vi "Navigation.vi"(0 "IA State Output in":T14, 1 "Penalty Shoot Out?":bool, 2 "PID gains Vel":T13={"proportional gain (Kc)"=0.6, "integral time (Ti, min)"=0.0, "derivative time (Td, min)"=0.0}, 3 "VelNearBall":dbl=1.0 format="%#_13g", 5 "Test Mode":bool, 6 "PID gains Angle":cluster{"(Kc)":dbl, "(Ki)":dbl, "(Kd)":dbl}={"(Kc)"=0.0, "(Ki)"=0.3, "(Kd)"=1.0}, 7 "a1":dbl=10.0, 8 "PID gains Lateral":cluster{"(Kc)":dbl, "(Ki)":dbl, "(Kd)":dbl}={"(Kc)"=2.0, "(Ki)"=0.0, "(Kd)"=0.3}, 9 "a3":dbl=15.0, 10 "Old GoTo Params":T12={"PID gains Angle GoTo"={"(Kc)"=3.0, "(Ki)"=0.0, "(Kd)"=2.0}, "PID gains XY GoTo"={"(Kc)"=3.0, "(Ki)"=0.0, "(Kd)"=2.0}, "Max Params GoTo"={"Max output XY"=3.0, "MaxOutput Angle"=0.0}}, 11 "GoTo Navigation":bool, 12 "Debug":bool, 13 "output inc":dbl, 14 "output xy":dbl, 15 "output angle":dbl) -> (4 "IA State Output out":T14)   [LabVIEW 2023]
uses:
  Vision_class/Old vision/SSL Detection Frame Simple Estimator Cameras VelCmd Folder/Core/AI Input.ctl
  Vision_class/Old vision/Controls/AI Robot.ctl
  Vision_class/Old vision/Controls/Functions Enum.ctl
  Controls/estimatives.ctl
  Vision_class/Old vision/Controls/AttackerStates.ctl
  Vision_class/Old vision/Controls/PathDests.ctl
  Vision_class/Old vision/Controls/PathDest.ctl
  VSSNavigation/VSSAttackerStates.ctl
  Robot_class/robotKickToStates.ctl
  Robot_class/roles.ctl
  <vilib>/Analysis/Matrix/Datatypes/RealMatrix.ctl
  driveMode.ctl
  Vision_class/Old vision/SSL Detection Frame Simple Estimator Cameras VelCmd Folder/Core/AI Ball.ctl
  Vision_class/Old vision/SSL Detection Frame Simple Estimator Cameras VelCmd Folder/Core/Field Size.ctl
  Vision_class/Old vision/SSL Detection Frame Simple Estimator Cameras VelCmd Folder/Core/AI Judge.ctl
  Communication_class/Paths/MessageAI_State Folder/Intel/Command Enum.ctl
  Vision_class/Old vision/SSL Detection Frame Simple Estimator Cameras VelCmd Folder/Util/Events/Events.ctl
  Utilities_class/Utilities.lvclass
  <vilib>/Analysis/Matrix/NI_Matrix.lvlib
panel:
  in  "Robot":T1={"id"=0, "function"=enum."Attacker", "x"=0.0, "y"=0.0, "orientation"=0.0, "v_tangent"=0.0, "v_normal"=0.0, "v_ang"=0.0, "kick_x"=0.0, "kick_z"=0.0, "dribble"=FALSE, "Timestamp"=timestamp(0 s since 1904-01-01), "estimatives"={"est_v_tangent"=0.0, "est_v_normal"=0.0, "est_vx"=0.0, "est_vy"=0.0, "Pos Robot Est"=[], "est_v_ang"=0.0}, "dest_x_kick"=0.0, "dest_y_kick"=0.0, "Gap Coord"=[], "States"=enum."GoToTangent", "Path "=[], "Path  Smooth"=[], "Dest"=[], "vx_desired"=0.0, "vy_desired"=0.0, "slowBehavior"=FALSE, "VSSStates"=enum."Pass", "robotKickState"=enum."none", "role"=enum."DefenderArea", "x_k|k"=[], "driveMode"=enum."Fast"}
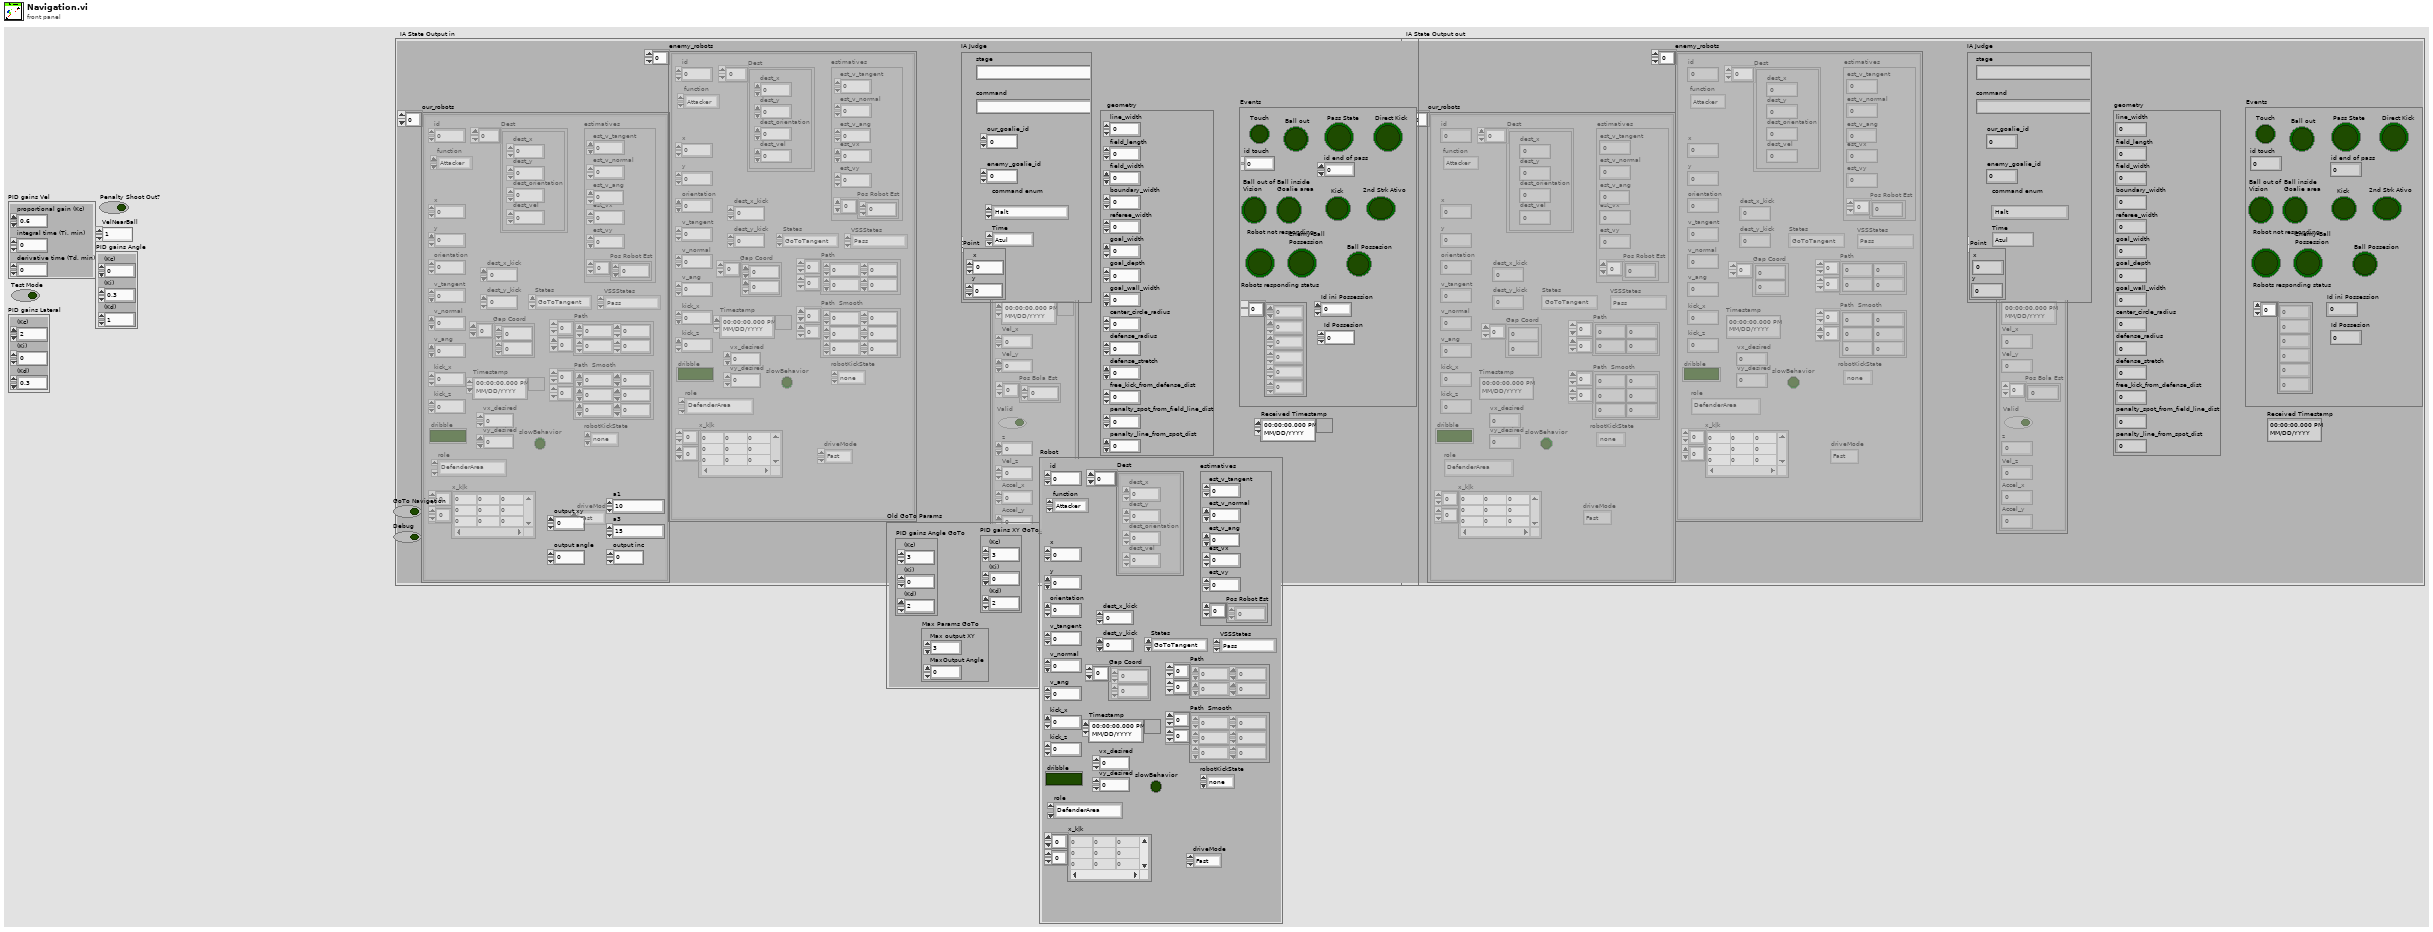
[diagram p1: front panel]
types:
  T1 = typedef "AI Robot.ctl" = cluster{"id":u32, "function":T2, "x":dbl, "y":dbl, "orientation":dbl, "v_tangent":dbl, "v_normal":dbl, "v_ang":dbl, "kick_x":dbl, "kick_z":dbl, "dribble":bool, "Timestamp":timestamp, "estimatives":T3, "dest_x_kick":dbl, "dest_y_kick":dbl, "Gap Coord":dbl[], "States":T4, "Path ":dbl[][], "Path  Smooth":dbl[][], "Dest":T5, "vx_desired":dbl, "vy_desired":dbl, "slowBehavior":bool, "VSSStates":T7, "robotKickState":T8, "role":T9, "x_k|k":T10, "driveMode":T11}
  T2 = typedef "Functions Enum.ctl" = enum16{"2nd Striker", "Attacker", "Goalie", "Defender", "Striker", "Goto 0", "Dummy", "Kicker", "ZigZag 0", "ZigZag 1", "ZigZag 2", "ZigZag 3", "ZigZag 4", "ZigZag 5", "ZigZag 6", "ZigZag 7", "ZigZag 8"}
  T3 = typedef "estimatives.ctl" = cluster{"est_v_tangent":dbl, "est_v_normal":dbl, "est_vx":dbl, "est_vy":dbl, "Pos Robot Est":dbl[], "est_v_ang":dbl}
  T4 = typedef "AttackerStates.ctl" = enum16{"Pass", "GoToTangent", "BallGetting", "GoToKick", ""}
  T5 = typedef "PathDests.ctl" = T6[]
  T6 = typedef "PathDest.ctl" = cluster{"dest_x":dbl, "dest_y":dbl, "dest_orientation":dbl, "dest_vel":dbl}
  T7 = typedef "VSSAttackerStates.ctl" = enum16{"Pass", "GoToTangent", "BallGetting", "GoToKick", "Rotate anti-clockwise", "Rotate Clockwise", ""}
  T8 = typedef "robotKickToStates.ctl" = enum16{"shootFromDirect", "avoidCollideBall", "goToBackBall", "none", "walk", "turn", "oldKickToShoot", "oldKickToGoToBackBall", "shoot"}
  T9 = typedef "roles.ctl" = enum16{"SimpleBallPlacement", "BallPlacementAllyPasser", "BallPlacementAllyReceiver", "BallPlacementEnemy", "5Robots5th", "PassBestReceiver", "5Robots4th", "5Robots3rd", "5Robots2nd", "5Robots1st", "PassBestRobot", "WaitPass", "ABCThirdKicker", "ABCFirstKicker", "ABCSecondKicker", "Tabler", "TableFinalizer", "PrepareRollToPassRoller", "PrepareRollToPassReceiver", "SimplePassRoll", "SimplePassRollReceiver", "PenaltyDefense", "PreparePassReceiver 2", "PreparePassReceiver 1", "PassObserver", "Timeout", "Goto", "ZigZag", "None", "BallOutOfField", "DefenderArea", "Duelist", "AttackerStop", "FollowAttacker", "KeeperRole", "KickPenalty", "AttackerAimGoal", "AttackerBlock", "Marker", "Halt", "Shoot", "PassKicker", "PassReceiver", "TestRole", "PenaltyAttacker", "PrimaryAttackerRole", "SupportAttackerRole"}
  T10 = typedef "NI_Matrix.lvlib/RealMatrix.ctl" = dbl[][]
  T11 = typedef "driveMode.ctl" = enum16{"Fast", "SafeDrive"}
  T12 = cluster{"PID gains Angle GoTo":cluster{"(Kc)":dbl, "(Ki)":dbl, "(Kd)":dbl}, "PID gains XY GoTo":cluster{"(Kc)":dbl, "(Ki)":dbl, "(Kd)":dbl}, "Max Params GoTo":cluster{"Max output XY":dbl, "MaxOutput Angle":dbl}}
  T13 = cluster{"proportional gain (Kc)":dbl, "integral time (Ti, min)":dbl, "derivative time (Td, min)":dbl}
  T14 = typedef "AI Input.ctl" = cluster{"our_robots":T1[], "enemy_robots":T1[], "balls":T15[], "geometry":T16, "IA Judge":T17, "Received Timestamp":timestamp, "Events":T19}
  T15 = typedef "AI Ball.ctl" = cluster{"x":dbl, "y":dbl, "timestamp":timestamp, "Vel_x":dbl, "Vel_y":dbl, "Pos Bola Est":dbl[], "Valid":bool, "z":dbl, "Vel_z":dbl, "Accel_x":dbl, "Accel_y":dbl}
  T16 = typedef "Field Size.ctl" = cluster{"line_width":u32, "field_length":u32, "field_width":u32, "boundary_width":u32, "referee_width":u32, "goal_width":u32, "goal_depth":u32, "goal_wall_width":u32, "center_circle_radius":u32, "defense_radius":u32, "defense_stretch":u32, "free_kick_from_defense_dist":u32, "penalty_spot_from_field_line_dist":u32, "penalty_line_from_spot_dist":u32}
  T17 = typedef "AI Judge.ctl" = cluster{"stage":string, "command":string, "our_goalie_id":dbl, "enemy_goalie_id":dbl, "command enum":T18, "Time":enum16{"Azul", "Amarelo"}, "Point":cluster{"x":sgl, "y":sgl}}
  T18 = typedef "Command Enum.ctl" = enum16{"Halt", "Stop", "Force Start", "PKA Normal Start", "Prepare Kickoff Ally", "PKE Normal Start", "Prepare Kickoff Enemy", "Prepare Penalty Ally", "PPA Normal Start", "Prepare Penalty Enemy", "PPE Normal Start", "Direct Free Enemy", "Direct Free Ally", "Indirect Free Enemy", "Indirect Free Ally", "Timeout Enemy", "Timeout Ally", "Goal Enemy", "Goal Ally", "Ball Placement Enemy", "Ball Placement Ally", "Normal Half Time", "Extra Time Break", "Extra Half Time", "None", "Post Game"}
  T19 = typedef "Events.ctl" = cluster{"Touch":bool, "Ball out":bool, "id touch":dbl, "Ball out of \nVision":bool, "Ball inside \nGoalie area":bool, "Robot not responding":bool, "Robots responding status":dbl[], "Enemy Ball \nPossession":bool, "Pass State":bool, "id end of pass":dbl, "Kick":bool, "Id ini Possession":dbl, "Ball Possesion":bool, "Id Possesion":dbl, "Direct Kick":bool, "2nd Strk Ativo":bool}
  T20 = cluster{"Max output XY":dbl, "MaxOutput Angle":dbl}
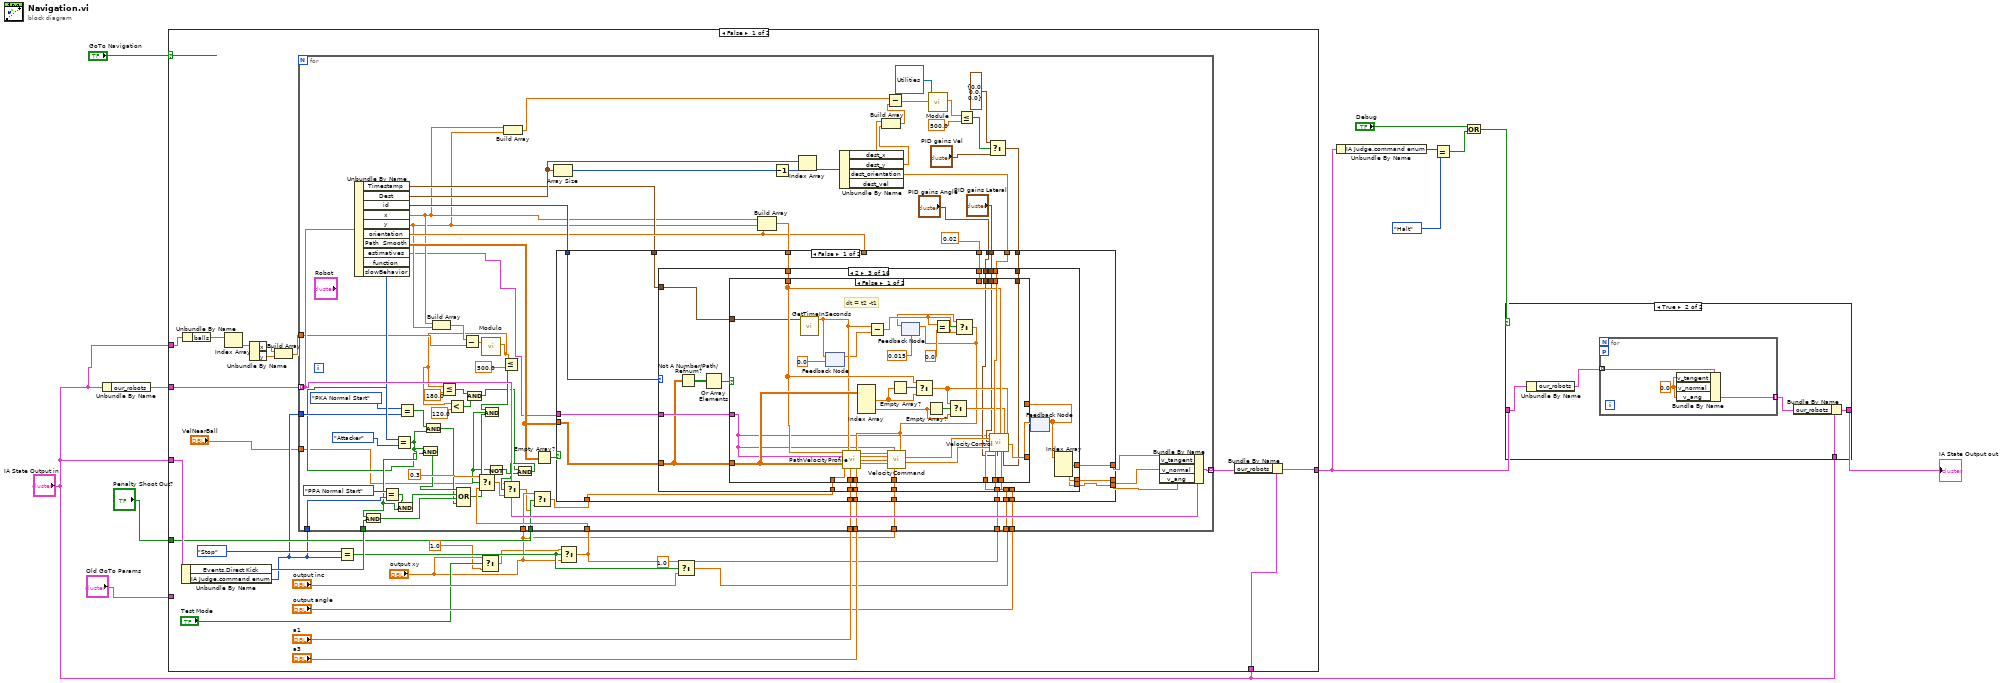
[diagram p0: block diagram]
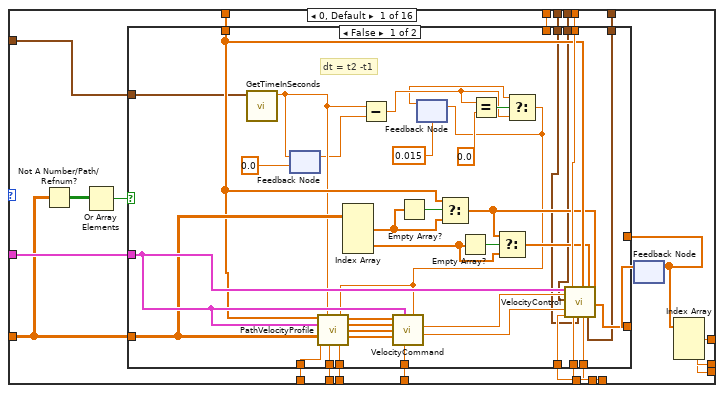
[diagram p2: hidden frame]
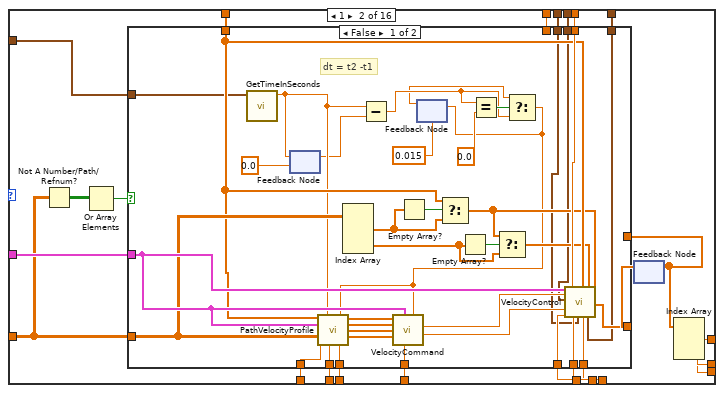
[diagram p4: hidden frame]
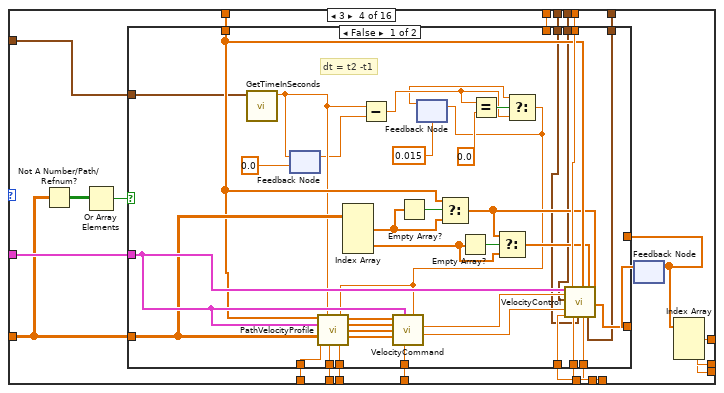
[diagram p7: hidden frame]
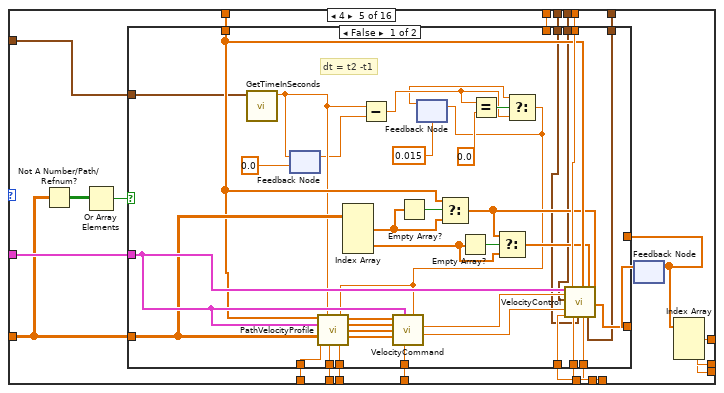
[diagram p9: hidden frame]
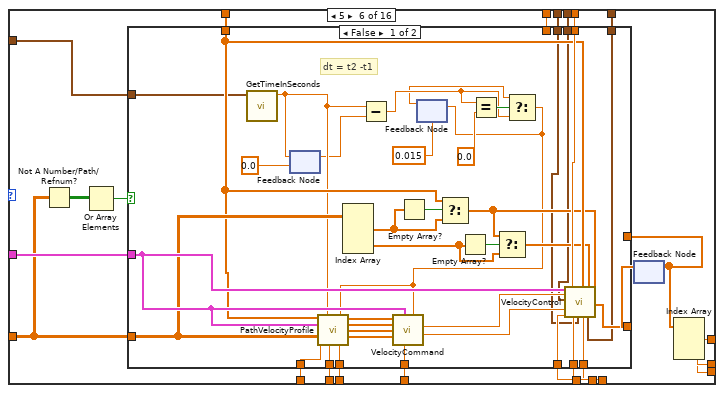
[diagram p11: hidden frame]
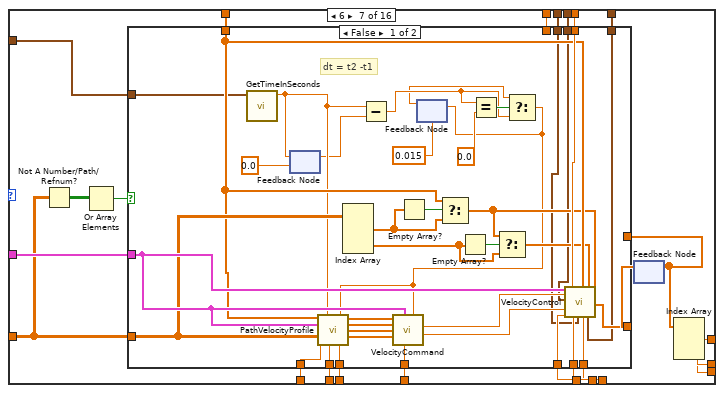
[diagram p13: hidden frame]
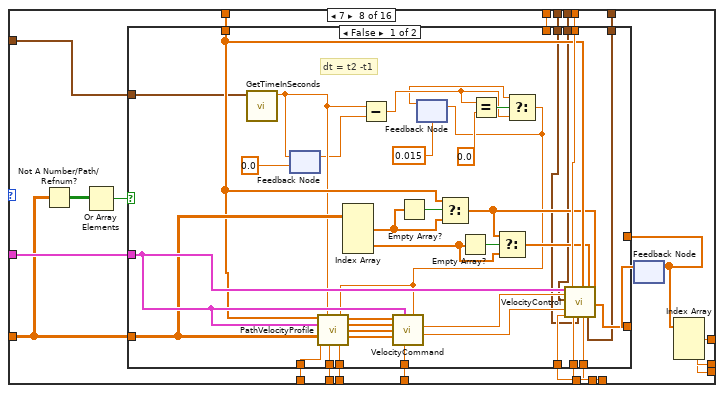
[diagram p15: hidden frame]
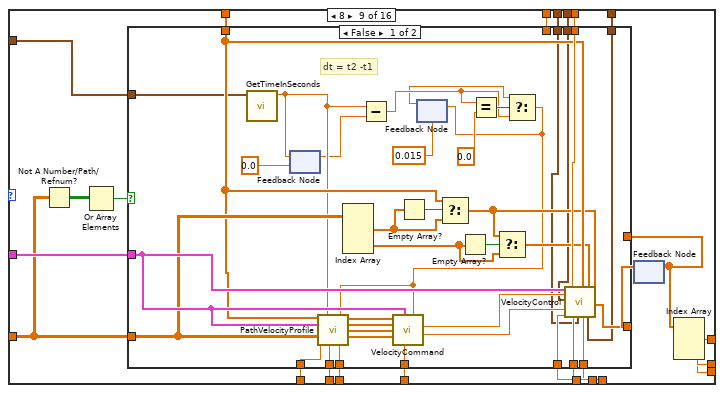
[diagram p17: hidden frame]
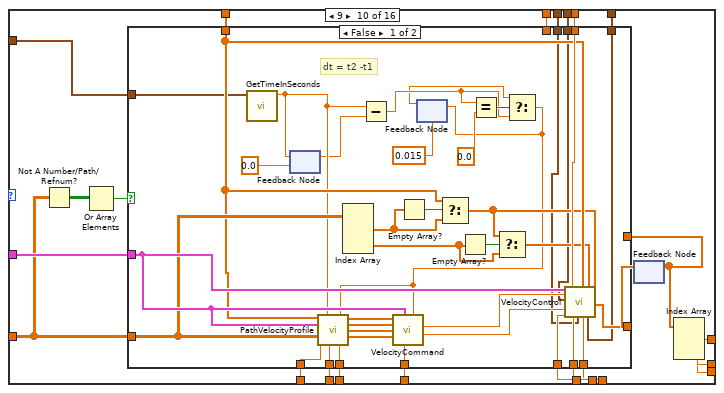
[diagram p19: hidden frame]
diagram:
  n1 = Unbundle By Name("IA State Output in") -> ("our_robots"=w12:T1[])
  n2 = case shown="False" "GoTo Navigation" {
    tunnel: w12 -> [w40 _]
    tunnel: [w37 w1121] -> w9
    tunnel: "IA State Output in" -> [w33 w1119]
    tunnel: "IA State Output in" -> [w38 _]
    tunnel: "IA State Output in" -> [w22 _]
    tunnel: "Penalty Shoot Out?" -> [w19 _]
    tunnel: "Old GoTo Params" -> [_ w1116]
    frame False {
      n3 = Unbundle By Name(w33) -> ("Events.Direct Kick"=w27:bool, "IA Judge.command enum"=w14:T18)
      n4 = Unbundle By Name(w22) -> ("balls"=w26:T15[])
      n5 = Index Array(array=w26) -> (element=w25:T15)  [unwired: 1 in]
      n6 = Unbundle By Name(w25) -> ("x"=w24:dbl, "y"=w23:dbl)
      n7 = Build Array(w24, w23) -> (w21:dbl[])
      n8 = Equal?(x=Command_Enum."Stop", y=w14) -> (x = y?=w20:bool)
      n9 = Select(t="output xy", s="Test Mode", f=1.0 ("t")) -> (s? t:f=w15:dbl)
      n10 = Select(t=w15, s=w20, f="output xy") -> (s? t:f=w31:dbl)
      n11 = Select(t=1.0, s=w20, f="output inc") -> (s? t:f=w29:dbl)
      n12 = for {
        tunnel: w40 -> [w118] mode=indexing
        tunnel: [w117] -> w39 mode=indexing
        tunnel: w31 -> [w96]
        tunnel: "a1" -> [w107]
        tunnel: "a3" -> [w106]
        tunnel: w29 -> [w102]
        tunnel: "output angle" -> [w101]
        tunnel: w31 -> [w100]
        tunnel: w14 -> [w94]
        tunnel: w27 -> [w88]
        tunnel: w14 -> [w86]
        tunnel: w21 -> [w77]
        tunnel: w19 -> [w74]
        tunnel: "output xy" -> [w73]
        tunnel: "output xy" -> [w58]
        tunnel: "VelNearBall" -> [w49]
        n13 = Unbundle By Name(w118) -> ("Timestamp"=w98:timestamp, "Dest"=w116:T5, "id"=w109:u32, "x"=w71:dbl, "y"=w70:dbl, "orientation"=w105:dbl, "Path  Smooth"=w110:dbl[][], "estimatives"=w46:T3, "function"=w87:T2, "slowBehavior"=w56:bool)
        n14 = Equal?(x=Command_Enum."PPA Normal Start", y=w94) -> (x = y?=w91:bool)
        n15 = Equal?(x=w87, y=Functions_Enum."Attacker") -> (x = y?=w83:bool)
        n16 = And(x=w83, y=w88) -> (x .and. y?=w89:bool)
        n17 = And(x=w91, y=w83) -> (x .and. y?=w90:bool)
        n18 = Equal?(x=Command_Enum."PKA Normal Start", y=w86) -> (x = y?=w84:bool)
        n19 = And(x=w83, y=w56) -> (x .and. y?=w92:bool)
        n20 = And(x=w84, y=w83) -> (x .and. y?=w82:bool)
        n21 = Build Array(w71, w70) -> (w78:dbl[])
        n22 = Compound Arithmetic op=OR(w92, w90, w89, w82) -> (w79:bool)
        n23 = Subtract(x=w78, y=w77) -> (x-y=w76:dbl[])
        n24 = call "Modulo.vi"("2D vector"=w76) -> ("Modulo"=w45:dbl)  [unwired: 10 in]
        n25 = Less Or Equal?(x=w45, y=180.0) -> (x <= y?=w43:bool)
        n26 = Less?(x=w45, y=120.0) -> (x < y?=w44:bool)
        n27 = And(x=w43, y=w44) -> (x .and. y?=w42:bool)
        n28 = Less Or Equal?(x=w45, y=500.0) -> (x <= y?=w80:bool)
        n29 = And(x=w80, y=w79) -> (x .and. y?=w54:bool)
        n30 = Select(t=0.3, s=w54, f=w96) -> (s? t:f=w51:dbl)
        n31 = Not(x=w54) -> (.not. x?=w53:bool)
        n32 = Build Array(w71, w70) -> (w66:dbl[])
        n33 = And(x=w42, y=w53) -> (x .and. y?=w52:bool)
        n34 = Select(t=w49, s=w52, f=w51) -> (s? t:f=w50:dbl)
        n35 = Select(t=w73, s=w74, f=w50) -> (s? t:f=w72:dbl)
        n36 = Empty Array?(array=w110) -> (empty?=w111:bool)
        n37 = Array Size(array=w116) -> (size(s)=w115:i32)
        n38 = Build Array(w71, w70, w105) -> (w108:dbl[])
        n39 = Decrement(x=w115) -> (x-1=w114:i32)
        n40 = Index Array(array=w116, index=w114) -> (element=w113:T6)
        n41 = Unbundle By Name(w113) -> ("dest_x"=w69:dbl, "dest_y"=w68:dbl, "dest_orientation"=w112:dbl)  [unwired: 1 out]
        n42 = Build Array(w69, w68) -> (w67:dbl[])
        n43 = Subtract(x=w66, y=w67) -> (x-y=w65:dbl[])
        n44 = call "Module.vi"("2D vector"=w65, "Utilities in"=refnum<class "Utilities.lvclass"> refnum) -> ("Modulo"=w63:dbl)  [unwired: 7 in, 2 out]
        n45 = Less Or Equal?(x=w63, y=500.0) -> (x <= y?=w61:bool)
        n46 = Select(t=T13 {"proportional gain (Kc)"=0.0, "integral time (Ti, min)"=0.0, "derivative time (Td, min)"=0.0}, s=w61, f="PID gains Vel") -> (s? t:f=w60:T13)
        n47 = case shown="False" w111 {
          tunnel: [w128 w1115] -> w104
          tunnel: [w127 w1115] -> w103
          tunnel: [w126 w1115] -> w99
          tunnel: w109 -> [w124 _]
          tunnel: w110 -> [w130 _]
          tunnel: w112 -> [w131 _]
          tunnel: w108 -> [w129 _]
          tunnel: w46 -> [w132 _]
          tunnel: w72 -> [w138 _]
          tunnel: w107 -> [w137 _]
          tunnel: w106 -> [w136 _]
          tunnel: w105 -> [_ _]
          tunnel: w102 -> [w135 _]
          tunnel: w101 -> [w134 _]
          tunnel: w100 -> [w133 _]
          tunnel: w98 -> [w125 _]
          tunnel: 0.02 -> [w123 _]
          tunnel: w60 -> [w122 _]
          tunnel: w58 -> [w121 _]
          tunnel: "PID gains Angle" -> [w120 _]
          tunnel: "PID gains Lateral" -> [w119 _]
          frame False {
            n48 = case shown="2" w124 {
              tunnel: w138 -> [w161 w222 w283 w344 w405 w466 w527 w588 w649 w710 w771 w832 w893 w954 w1015 w1076]
              tunnel: w137 -> [w160 w221 w282 w343 w404 w465 w526 w587 w648 w709 w770 w831 w892 w953 w1014 w1075]
              tunnel: w136 -> [w159 w220 w281 w342 w403 w464 w525 w586 w647 w708 w769 w830 w891 w952 w1013 w1074]
              tunnel: w135 -> [w158 w219 w280 w341 w402 w463 w524 w585 w646 w707 w768 w829 w890 w951 w1012 w1073]
              tunnel: w134 -> [w157 w218 w279 w340 w401 w462 w523 w584 w645 w706 w767 w828 w889 w950 w1011 w1072]
              tunnel: w133 -> [w156 w217 w278 w339 w400 w461 w522 w583 w644 w705 w766 w827 w888 w949 w1010 w1071]
              tunnel: w132 -> [w155 w216 w277 w338 w399 w460 w521 w582 w643 w704 w765 w826 w887 w948 w1009 w1070]
              tunnel: w131 -> [w154 w215 w276 w337 w398 w459 w520 w581 w642 w703 w764 w825 w886 w947 w1008 w1069]
              tunnel: w130 -> [w146 w207 w268 w329 w390 w451 w512 w573 w634 w695 w756 w817 w878 w939 w1000 w1061]
              tunnel: w129 -> [w153 w214 w275 w336 w397 w458 w519 w580 w641 w702 w763 w824 w885 w946 w1007 w1068]
              tunnel: [w152 w213 w274 w335 w396 w457 w518 w579 w640 w701 w762 w823 w884 w945 w1006 w1067] -> w128
              tunnel: [w151 w212 w273 w334 w395 w456 w517 w578 w639 w700 w761 w822 w883 w944 w1005 w1066] -> w127
              tunnel: [w150 w211 w272 w333 w394 w455 w516 w577 w638 w699 w760 w821 w882 w943 w1004 w1065] -> w126
              tunnel: w125 -> [w149 w210 w271 w332 w393 w454 w515 w576 w637 w698 w759 w820 w881 w942 w1003 w1064]
              tunnel: w123 -> [w143 w204 w265 w326 w387 w448 w509 w570 w631 w692 w753 w814 w875 w936 w997 w1058]
              tunnel: w122 -> [w142 w203 w264 w325 w386 w447 w508 w569 w630 w691 w752 w813 w874 w935 w996 w1057]
              tunnel: w121 -> [w141 w202 w263 w324 w385 w446 w507 w568 w629 w690 w751 w812 w873 w934 w995 w1056]
              tunnel: w120 -> [w140 w201 w262 w323 w384 w445 w506 w567 w628 w689 w750 w811 w872 w933 w994 w1055]
              tunnel: w119 -> [w139 w200 w261 w322 w383 w444 w505 w566 w627 w688 w749 w810 w871 w932 w993 w1054]
              frame 0, Default {
                n49 = Not A Number/Path/Refnum?(number/path/refnum=w146) -> (NaN/Path/Refnum?=w145:bool[][])
                n50 = Or Array Elements(Boolean array=w145) -> (logical OR=w144:bool)
                n51 = feedback #1() -> (w147:dbl[])  [unwired: 1 in]
                n52 = case shown="False" w144 {
                  tunnel: w161 -> [w198 _]
                  tunnel: w160 -> [w197 _]
                  tunnel: w159 -> [w196 _]
                  tunnel: w158 -> [w195 _]
                  tunnel: w157 -> [w194 _]
                  tunnel: w156 -> [w193 _]
                  tunnel: w155 -> [w192 _]
                  tunnel: w154 -> [w191 _]
                  tunnel: w146 -> [w190 _]
                  tunnel: w153 -> [w189 _]
                  tunnel: [w188 w199] -> w148
                  tunnel: w149 -> [w175 _]
                  tunnel: w147 -> [_ w199]
                  tunnel: w143 -> [_ _]
                  tunnel: w142 -> [w166 _]
                  tunnel: w141 -> [w164 _]
                  tunnel: w140 -> [w163 _]
                  tunnel: w139 -> [w162 _]
                  frame False {
                    # "dt = t2 -t1"
                    n53 = call "GetTimeInSeconds.vi"("Timestamp"=w175) -> ("Numeric"=w169:dbl)  [unwired: 10 in]
                    n54 = feedback-in #2(w169) -> ()
                    n55 = feedback #2(0.0 ("Numeric")) -> (w168:dbl)
                    n56 = Index Array(array=w190) -> (element #1=w177:dbl[], element #2=w180:dbl[])  [unwired: 4 in]
                    n57 = Subtract(x=w169, y=w168) -> (x-y=w171:dbl)
                    n58 = Empty Array?(array=w177) -> (empty?=w178:bool)
                    n59 = feedback #3(0.015 ("Numeric")) -> (w170:dbl)
                    n60 = Select(t=w189, s=w178, f=w177) -> (s? t:f=w176:dbl[])
                    n61 = Empty Array?(array=w180) -> (empty?=w181:bool)
                    n62 = Equal?(x=w171, y=0.0) -> (x = y?=w174:bool)
                    n63 = Select(t=w176, s=w181, f=w180) -> (s? t:f=w179:dbl[])
                    n64 = Select(t=w170, s=w174, f=w171) -> (s? t:f=w165:dbl)
                    n65 = call "PathVelocityProfile.vi"("Pose"=w189, "time"=w169, "intervalo"=w165, "estimatives"=w192, "Path  Smooth"=w190, "V_max"=w198, "Accel"=w197, "DesAccel"=w196) -> ("Time X"=w187:dbl[], "Velocities X"=w186:dbl[], "Time Y"=w185:dbl[], "Velocities Y"=w184:dbl[])  [unwired: 4 in]
                    n66 = call "VelocityCommand.vi"("intervalo"=w165, "MaxOutputXY"=w164, "estimatives"=w192, "Velocities Y"=w184, "Time Y"=w185, "Velocities X"=w186, "Time X"=w187) -> ("Vy"=w183:dbl, "Vx"=w182:dbl)  [unwired: 3 in]
                    n67 = feedback-in #3(w165) -> ()
                    n68 = call "VelocityControl.vi"("estimatives"=w192, "Vx"=w182, "PID Gains lateral"=w162, "Vy"=w183, "output xy"=w193, "Dest_orientation"=w191, "output inc"=w195, "PID Gains Angle"=w163, "Position"=w189, "output angle"=w194, "Waypoint 1"=w179, "PID gains Vel"=w166, "Waypoint 0"=w176) -> ("Output Velocity"=w188:dbl[])  [unwired: 6 in]
                  }
                  frame True {
                  }
                }
                n69 = feedback-in #1(w148) -> ()
                n70 = Index Array(array=w147) -> (element #1=w152:dbl, element #2=w151:dbl, element #3=w150:dbl)  [unwired: 3 in]
              }
              frame 1 {
                n71 = Not A Number/Path/Refnum?(number/path/refnum=w207) -> (NaN/Path/Refnum?=w206:bool[][])
                n72 = Or Array Elements(Boolean array=w206) -> (logical OR=w205:bool)
                n73 = feedback #4() -> (w208:dbl[])  [unwired: 1 in]
                n74 = case shown="False" w205 {
                  tunnel: w222 -> [w259 _]
                  tunnel: w221 -> [w258 _]
                  tunnel: w220 -> [w257 _]
                  tunnel: w219 -> [w256 _]
                  tunnel: w218 -> [w255 _]
                  tunnel: w217 -> [w254 _]
                  tunnel: w216 -> [w253 _]
                  tunnel: w215 -> [w252 _]
                  tunnel: w207 -> [w251 _]
                  tunnel: w214 -> [w250 _]
                  tunnel: [w249 w260] -> w209
                  tunnel: w210 -> [w236 _]
                  tunnel: w208 -> [_ w260]
                  tunnel: w204 -> [_ _]
                  tunnel: w203 -> [w227 _]
                  tunnel: w202 -> [w225 _]
                  tunnel: w201 -> [w224 _]
                  tunnel: w200 -> [w223 _]
                  frame False {
                    # "dt = t2 -t1"
                    n75 = call "GetTimeInSeconds.vi"("Timestamp"=w236) -> ("Numeric"=w230:dbl)  [unwired: 10 in]
                    n76 = feedback-in #5(w230) -> ()
                    n77 = feedback #5(0.0 ("Numeric")) -> (w229:dbl)
                    n78 = Index Array(array=w251) -> (element #1=w238:dbl[], element #2=w241:dbl[])  [unwired: 4 in]
                    n79 = Subtract(x=w230, y=w229) -> (x-y=w232:dbl)
                    n80 = Empty Array?(array=w238) -> (empty?=w239:bool)
                    n81 = feedback #6(0.015 ("Numeric")) -> (w231:dbl)
                    n82 = Select(t=w250, s=w239, f=w238) -> (s? t:f=w237:dbl[])
                    n83 = Empty Array?(array=w241) -> (empty?=w242:bool)
                    n84 = Equal?(x=w232, y=0.0) -> (x = y?=w235:bool)
                    n85 = Select(t=w237, s=w242, f=w241) -> (s? t:f=w240:dbl[])
                    n86 = Select(t=w231, s=w235, f=w232) -> (s? t:f=w226:dbl)
                    n87 = call "PathVelocityProfile.vi"("Pose"=w250, "time"=w230, "intervalo"=w226, "estimatives"=w253, "Path  Smooth"=w251, "V_max"=w259, "Accel"=w258, "DesAccel"=w257) -> ("Time X"=w248:dbl[], "Velocities X"=w247:dbl[], "Time Y"=w246:dbl[], "Velocities Y"=w245:dbl[])  [unwired: 4 in]
                    n88 = call "VelocityCommand.vi"("intervalo"=w226, "MaxOutputXY"=w225, "estimatives"=w253, "Velocities Y"=w245, "Time Y"=w246, "Velocities X"=w247, "Time X"=w248) -> ("Vy"=w244:dbl, "Vx"=w243:dbl)  [unwired: 3 in]
                    n89 = feedback-in #6(w226) -> ()
                    n90 = call "VelocityControl.vi"("estimatives"=w253, "Vx"=w243, "PID Gains lateral"=w223, "Vy"=w244, "output xy"=w254, "Dest_orientation"=w252, "output inc"=w256, "PID Gains Angle"=w224, "Position"=w250, "output angle"=w255, "Waypoint 1"=w240, "PID gains Vel"=w227, "Waypoint 0"=w237) -> ("Output Velocity"=w249:dbl[])  [unwired: 6 in]
                  }
                  frame True {
                  }
                }
                n91 = feedback-in #4(w209) -> ()
                n92 = Index Array(array=w208) -> (element #1=w213:dbl, element #2=w212:dbl, element #3=w211:dbl)  [unwired: 3 in]
              }
              frame 2 {
                n93 = Not A Number/Path/Refnum?(number/path/refnum=w268) -> (NaN/Path/Refnum?=w267:bool[][])
                n94 = Or Array Elements(Boolean array=w267) -> (logical OR=w266:bool)
                n95 = feedback #7() -> (w269:dbl[])  [unwired: 1 in]
                n96 = case shown="False" w266 {
                  tunnel: w283 -> [w320 _]
                  tunnel: w282 -> [w319 _]
                  tunnel: w281 -> [w318 _]
                  tunnel: w280 -> [w317 _]
                  tunnel: w279 -> [w316 _]
                  tunnel: w278 -> [w315 _]
                  tunnel: w277 -> [w284 _]
                  tunnel: w276 -> [w314 _]
                  tunnel: w268 -> [w313 _]
                  tunnel: w275 -> [w312 _]
                  tunnel: [w311 w321] -> w270
                  tunnel: w271 -> [w298 _]
                  tunnel: w269 -> [_ w321]
                  tunnel: w265 -> [_ _]
                  tunnel: w264 -> [w289 _]
                  tunnel: w263 -> [w287 _]
                  tunnel: w262 -> [w286 _]
                  tunnel: w261 -> [w285 _]
                  frame False {
                    # "dt = t2 -t1"
                    n97 = call "GetTimeInSeconds.vi"("Timestamp"=w298) -> ("Numeric"=w292:dbl)  [unwired: 10 in]
                    n98 = feedback-in #8(w292) -> ()
                    n99 = feedback #8(0.0 ("Numeric")) -> (w291:dbl)
                    n100 = Index Array(array=w313) -> (element #1=w300:dbl[], element #2=w303:dbl[])  [unwired: 4 in]
                    n101 = Subtract(x=w292, y=w291) -> (x-y=w294:dbl)
                    n102 = Empty Array?(array=w300) -> (empty?=w301:bool)
                    n103 = feedback #9(0.015 ("Numeric")) -> (w293:dbl)
                    n104 = Select(t=w312, s=w301, f=w300) -> (s? t:f=w299:dbl[])
                    n105 = Empty Array?(array=w303) -> (empty?=w304:bool)
                    n106 = Equal?(x=w294, y=0.0) -> (x = y?=w297:bool)
                    n107 = Select(t=w299, s=w304, f=w303) -> (s? t:f=w302:dbl[])
                    n108 = Select(t=w293, s=w297, f=w294) -> (s? t:f=w288:dbl)
                    n109 = call "PathVelocityProfile.vi"("Pose"=w312, "time"=w292, "intervalo"=w288, "estimatives"=w284, "Path  Smooth"=w313, "V_max"=w320, "Accel"=w319, "DesAccel"=w318) -> ("Time X"=w310:dbl[], "Velocities X"=w309:dbl[], "Time Y"=w308:dbl[], "Velocities Y"=w307:dbl[])  [unwired: 4 in]
                    n110 = call "VelocityCommand.vi"("intervalo"=w288, "MaxOutputXY"=w287, "estimatives"=w284, "Velocities Y"=w307, "Time Y"=w308, "Velocities X"=w309, "Time X"=w310) -> ("Vy"=w306:dbl, "Vx"=w305:dbl)  [unwired: 3 in]
                    n111 = feedback-in #9(w288) -> ()
                    n112 = call "VelocityControl.vi"("estimatives"=w284, "Vx"=w305, "PID Gains lateral"=w285, "Vy"=w306, "output xy"=w315, "Dest_orientation"=w314, "output inc"=w317, "PID Gains Angle"=w286, "Position"=w312, "output angle"=w316, "Waypoint 1"=w302, "PID gains Vel"=w289, "Waypoint 0"=w299) -> ("Output Velocity"=w311:dbl[])  [unwired: 6 in]
                  }
                  frame True {
                  }
                }
                n113 = feedback-in #7(w270) -> ()
                n114 = Index Array(array=w269) -> (element #1=w274:dbl, element #2=w273:dbl, element #3=w272:dbl)  [unwired: 3 in]
              }
              frame 3 {
                n115 = Not A Number/Path/Refnum?(number/path/refnum=w329) -> (NaN/Path/Refnum?=w328:bool[][])
                n116 = Or Array Elements(Boolean array=w328) -> (logical OR=w327:bool)
                n117 = feedback #10() -> (w330:dbl[])  [unwired: 1 in]
                n118 = case shown="False" w327 {
                  tunnel: w344 -> [w381 _]
                  tunnel: w343 -> [w380 _]
                  tunnel: w342 -> [w379 _]
                  tunnel: w341 -> [w378 _]
                  tunnel: w340 -> [w377 _]
                  tunnel: w339 -> [w376 _]
                  tunnel: w338 -> [w375 _]
                  tunnel: w337 -> [w374 _]
                  tunnel: w329 -> [w373 _]
                  tunnel: w336 -> [w372 _]
                  tunnel: [w371 w382] -> w331
                  tunnel: w332 -> [w358 _]
                  tunnel: w330 -> [_ w382]
                  tunnel: w326 -> [_ _]
                  tunnel: w325 -> [w349 _]
                  tunnel: w324 -> [w347 _]
                  tunnel: w323 -> [w346 _]
                  tunnel: w322 -> [w345 _]
                  frame False {
                    # "dt = t2 -t1"
                    n119 = call "GetTimeInSeconds.vi"("Timestamp"=w358) -> ("Numeric"=w352:dbl)  [unwired: 10 in]
                    n120 = feedback-in #11(w352) -> ()
                    n121 = feedback #11(0.0 ("Numeric")) -> (w351:dbl)
                    n122 = Index Array(array=w373) -> (element #1=w360:dbl[], element #2=w363:dbl[])  [unwired: 4 in]
                    n123 = Subtract(x=w352, y=w351) -> (x-y=w354:dbl)
                    n124 = Empty Array?(array=w360) -> (empty?=w361:bool)
                    n125 = feedback #12(0.015 ("Numeric")) -> (w353:dbl)
                    n126 = Select(t=w372, s=w361, f=w360) -> (s? t:f=w359:dbl[])
                    n127 = Empty Array?(array=w363) -> (empty?=w364:bool)
                    n128 = Equal?(x=w354, y=0.0) -> (x = y?=w357:bool)
                    n129 = Select(t=w359, s=w364, f=w363) -> (s? t:f=w362:dbl[])
                    n130 = Select(t=w353, s=w357, f=w354) -> (s? t:f=w348:dbl)
                    n131 = call "PathVelocityProfile.vi"("Pose"=w372, "time"=w352, "intervalo"=w348, "estimatives"=w375, "Path  Smooth"=w373, "V_max"=w381, "Accel"=w380, "DesAccel"=w379) -> ("Time X"=w370:dbl[], "Velocities X"=w369:dbl[], "Time Y"=w368:dbl[], "Velocities Y"=w367:dbl[])  [unwired: 4 in]
                    n132 = call "VelocityCommand.vi"("intervalo"=w348, "MaxOutputXY"=w347, "estimatives"=w375, "Velocities Y"=w367, "Time Y"=w368, "Velocities X"=w369, "Time X"=w370) -> ("Vy"=w366:dbl, "Vx"=w365:dbl)  [unwired: 3 in]
                    n133 = feedback-in #12(w348) -> ()
                    n134 = call "VelocityControl.vi"("estimatives"=w375, "Vx"=w365, "PID Gains lateral"=w345, "Vy"=w366, "output xy"=w376, "Dest_orientation"=w374, "output inc"=w378, "PID Gains Angle"=w346, "Position"=w372, "output angle"=w377, "Waypoint 1"=w362, "PID gains Vel"=w349, "Waypoint 0"=w359) -> ("Output Velocity"=w371:dbl[])  [unwired: 6 in]
                  }
                  frame True {
                  }
                }
                n135 = feedback-in #10(w331) -> ()
                n136 = Index Array(array=w330) -> (element #1=w335:dbl, element #2=w334:dbl, element #3=w333:dbl)  [unwired: 3 in]
              }
              frame 4 {
                n137 = Not A Number/Path/Refnum?(number/path/refnum=w390) -> (NaN/Path/Refnum?=w389:bool[][])
                n138 = Or Array Elements(Boolean array=w389) -> (logical OR=w388:bool)
                n139 = feedback #13() -> (w391:dbl[])  [unwired: 1 in]
                n140 = case shown="False" w388 {
                  tunnel: w405 -> [w442 _]
                  tunnel: w404 -> [w441 _]
                  tunnel: w403 -> [w440 _]
                  tunnel: w402 -> [w439 _]
                  tunnel: w401 -> [w438 _]
                  tunnel: w400 -> [w437 _]
                  tunnel: w399 -> [w436 _]
                  tunnel: w398 -> [w435 _]
                  tunnel: w390 -> [w434 _]
                  tunnel: w397 -> [w433 _]
                  tunnel: [w432 w443] -> w392
                  tunnel: w393 -> [w419 _]
                  tunnel: w391 -> [_ w443]
                  tunnel: w387 -> [_ _]
                  tunnel: w386 -> [w410 _]
                  tunnel: w385 -> [w408 _]
                  tunnel: w384 -> [w407 _]
                  tunnel: w383 -> [w406 _]
                  frame False {
                    # "dt = t2 -t1"
                    n141 = call "GetTimeInSeconds.vi"("Timestamp"=w419) -> ("Numeric"=w413:dbl)  [unwired: 10 in]
                    n142 = feedback-in #14(w413) -> ()
                    n143 = feedback #14(0.0 ("Numeric")) -> (w412:dbl)
                    n144 = Index Array(array=w434) -> (element #1=w421:dbl[], element #2=w424:dbl[])  [unwired: 4 in]
                    n145 = Subtract(x=w413, y=w412) -> (x-y=w415:dbl)
                    n146 = Empty Array?(array=w421) -> (empty?=w422:bool)
                    n147 = feedback #15(0.015 ("Numeric")) -> (w414:dbl)
                    n148 = Select(t=w433, s=w422, f=w421) -> (s? t:f=w420:dbl[])
                    n149 = Empty Array?(array=w424) -> (empty?=w425:bool)
                    n150 = Equal?(x=w415, y=0.0) -> (x = y?=w418:bool)
                    n151 = Select(t=w420, s=w425, f=w424) -> (s? t:f=w423:dbl[])
                    n152 = Select(t=w414, s=w418, f=w415) -> (s? t:f=w409:dbl)
                    n153 = call "PathVelocityProfile.vi"("Pose"=w433, "time"=w413, "intervalo"=w409, "estimatives"=w436, "Path  Smooth"=w434, "V_max"=w442, "Accel"=w441, "DesAccel"=w440) -> ("Time X"=w431:dbl[], "Velocities X"=w430:dbl[], "Time Y"=w429:dbl[], "Velocities Y"=w428:dbl[])  [unwired: 4 in]
                    n154 = call "VelocityCommand.vi"("intervalo"=w409, "MaxOutputXY"=w408, "estimatives"=w436, "Velocities Y"=w428, "Time Y"=w429, "Velocities X"=w430, "Time X"=w431) -> ("Vy"=w427:dbl, "Vx"=w426:dbl)  [unwired: 3 in]
                    n155 = feedback-in #15(w409) -> ()
                    n156 = call "VelocityControl.vi"("estimatives"=w436, "Vx"=w426, "PID Gains lateral"=w406, "Vy"=w427, "output xy"=w437, "Dest_orientation"=w435, "output inc"=w439, "PID Gains Angle"=w407, "Position"=w433, "output angle"=w438, "Waypoint 1"=w423, "PID gains Vel"=w410, "Waypoint 0"=w420) -> ("Output Velocity"=w432:dbl[])  [unwired: 6 in]
                  }
                  frame True {
                  }
                }
                n157 = feedback-in #13(w392) -> ()
                n158 = Index Array(array=w391) -> (element #1=w396:dbl, element #2=w395:dbl, element #3=w394:dbl)  [unwired: 3 in]
              }
              frame 5 {
                n159 = Not A Number/Path/Refnum?(number/path/refnum=w451) -> (NaN/Path/Refnum?=w450:bool[][])
                n160 = Or Array Elements(Boolean array=w450) -> (logical OR=w449:bool)
                n161 = feedback #16() -> (w452:dbl[])  [unwired: 1 in]
                n162 = case shown="False" w449 {
                  tunnel: w466 -> [w503 _]
                  tunnel: w465 -> [w502 _]
                  tunnel: w464 -> [w501 _]
                  tunnel: w463 -> [w500 _]
                  tunnel: w462 -> [w499 _]
                  tunnel: w461 -> [w498 _]
                  tunnel: w460 -> [w497 _]
                  tunnel: w459 -> [w496 _]
                  tunnel: w451 -> [w495 _]
                  tunnel: w458 -> [w494 _]
                  tunnel: [w493 w504] -> w453
                  tunnel: w454 -> [w480 _]
                  tunnel: w452 -> [_ w504]
                  tunnel: w448 -> [_ _]
                  tunnel: w447 -> [w471 _]
                  tunnel: w446 -> [w469 _]
                  tunnel: w445 -> [w468 _]
                  tunnel: w444 -> [w467 _]
                  frame False {
                    # "dt = t2 -t1"
                    n163 = call "GetTimeInSeconds.vi"("Timestamp"=w480) -> ("Numeric"=w474:dbl)  [unwired: 10 in]
                    n164 = feedback-in #17(w474) -> ()
                    n165 = feedback #17(0.0 ("Numeric")) -> (w473:dbl)
                    n166 = Index Array(array=w495) -> (element #1=w482:dbl[], element #2=w485:dbl[])  [unwired: 4 in]
                    n167 = Subtract(x=w474, y=w473) -> (x-y=w476:dbl)
                    n168 = Empty Array?(array=w482) -> (empty?=w483:bool)
                    n169 = feedback #18(0.015 ("Numeric")) -> (w475:dbl)
                    n170 = Select(t=w494, s=w483, f=w482) -> (s? t:f=w481:dbl[])
                    n171 = Empty Array?(array=w485) -> (empty?=w486:bool)
                    n172 = Equal?(x=w476, y=0.0) -> (x = y?=w479:bool)
                    n173 = Select(t=w481, s=w486, f=w485) -> (s? t:f=w484:dbl[])
                    n174 = Select(t=w475, s=w479, f=w476) -> (s? t:f=w470:dbl)
                    n175 = call "PathVelocityProfile.vi"("Pose"=w494, "time"=w474, "intervalo"=w470, "estimatives"=w497, "Path  Smooth"=w495, "V_max"=w503, "Accel"=w502, "DesAccel"=w501) -> ("Time X"=w492:dbl[], "Velocities X"=w491:dbl[], "Time Y"=w490:dbl[], "Velocities Y"=w489:dbl[])  [unwired: 4 in]
                    n176 = call "VelocityCommand.vi"("intervalo"=w470, "MaxOutputXY"=w469, "estimatives"=w497, "Velocities Y"=w489, "Time Y"=w490, "Velocities X"=w491, "Time X"=w492) -> ("Vy"=w488:dbl, "Vx"=w487:dbl)  [unwired: 3 in]
                    n177 = feedback-in #18(w470) -> ()
                    n178 = call "VelocityControl.vi"("estimatives"=w497, "Vx"=w487, "PID Gains lateral"=w467, "Vy"=w488, "output xy"=w498, "Dest_orientation"=w496, "output inc"=w500, "PID Gains Angle"=w468, "Position"=w494, "output angle"=w499, "Waypoint 1"=w484, "PID gains Vel"=w471, "Waypoint 0"=w481) -> ("Output Velocity"=w493:dbl[])  [unwired: 6 in]
                  }
                  frame True {
                  }
                }
                n179 = feedback-in #16(w453) -> ()
                n180 = Index Array(array=w452) -> (element #1=w457:dbl, element #2=w456:dbl, element #3=w455:dbl)  [unwired: 3 in]
              }
              frame 6 {
                n181 = Not A Number/Path/Refnum?(number/path/refnum=w512) -> (NaN/Path/Refnum?=w511:bool[][])
                n182 = Or Array Elements(Boolean array=w511) -> (logical OR=w510:bool)
                n183 = feedback #19() -> (w513:dbl[])  [unwired: 1 in]
                n184 = case shown="False" w510 {
                  tunnel: w527 -> [w564 _]
                  tunnel: w526 -> [w563 _]
                  tunnel: w525 -> [w562 _]
                  tunnel: w524 -> [w561 _]
                  tunnel: w523 -> [w560 _]
                  tunnel: w522 -> [w559 _]
                  tunnel: w521 -> [w558 _]
                  tunnel: w520 -> [w557 _]
                  tunnel: w512 -> [w556 _]
                  tunnel: w519 -> [w555 _]
                  tunnel: [w554 w565] -> w514
                  tunnel: w515 -> [w541 _]
                  tunnel: w513 -> [_ w565]
                  tunnel: w509 -> [_ _]
                  tunnel: w508 -> [w532 _]
                  tunnel: w507 -> [w530 _]
                  tunnel: w506 -> [w529 _]
                  tunnel: w505 -> [w528 _]
                  frame False {
                    # "dt = t2 -t1"
                    n185 = call "GetTimeInSeconds.vi"("Timestamp"=w541) -> ("Numeric"=w535:dbl)  [unwired: 10 in]
                    n186 = feedback-in #20(w535) -> ()
                    n187 = feedback #20(0.0 ("Numeric")) -> (w534:dbl)
                    n188 = Index Array(array=w556) -> (element #1=w543:dbl[], element #2=w546:dbl[])  [unwired: 4 in]
                    n189 = Subtract(x=w535, y=w534) -> (x-y=w537:dbl)
                    n190 = Empty Array?(array=w543) -> (empty?=w544:bool)
                    n191 = feedback #21(0.015 ("Numeric")) -> (w536:dbl)
                    n192 = Select(t=w555, s=w544, f=w543) -> (s? t:f=w542:dbl[])
                    n193 = Empty Array?(array=w546) -> (empty?=w547:bool)
                    n194 = Equal?(x=w537, y=0.0) -> (x = y?=w540:bool)
                    n195 = Select(t=w542, s=w547, f=w546) -> (s? t:f=w545:dbl[])
                    n196 = Select(t=w536, s=w540, f=w537) -> (s? t:f=w531:dbl)
                    n197 = call "PathVelocityProfile.vi"("Pose"=w555, "time"=w535, "intervalo"=w531, "estimatives"=w558, "Path  Smooth"=w556, "V_max"=w564, "Accel"=w563, "DesAccel"=w562) -> ("Time X"=w553:dbl[], "Velocities X"=w552:dbl[], "Time Y"=w551:dbl[], "Velocities Y"=w550:dbl[])  [unwired: 4 in]
                    n198 = call "VelocityCommand.vi"("intervalo"=w531, "MaxOutputXY"=w530, "estimatives"=w558, "Velocities Y"=w550, "Time Y"=w551, "Velocities X"=w552, "Time X"=w553) -> ("Vy"=w549:dbl, "Vx"=w548:dbl)  [unwired: 3 in]
                    n199 = feedback-in #21(w531) -> ()
                    n200 = call "VelocityControl.vi"("estimatives"=w558, "Vx"=w548, "PID Gains lateral"=w528, "Vy"=w549, "output xy"=w559, "Dest_orientation"=w557, "output inc"=w561, "PID Gains Angle"=w529, "Position"=w555, "output angle"=w560, "Waypoint 1"=w545, "PID gains Vel"=w532, "Waypoint 0"=w542) -> ("Output Velocity"=w554:dbl[])  [unwired: 6 in]
                  }
                  frame True {
                  }
                }
                n201 = feedback-in #19(w514) -> ()
                n202 = Index Array(array=w513) -> (element #1=w518:dbl, element #2=w517:dbl, element #3=w516:dbl)  [unwired: 3 in]
              }
              frame 7 {
                n203 = Not A Number/Path/Refnum?(number/path/refnum=w573) -> (NaN/Path/Refnum?=w572:bool[][])
                n204 = Or Array Elements(Boolean array=w572) -> (logical OR=w571:bool)
                n205 = feedback #22() -> (w574:dbl[])  [unwired: 1 in]
                n206 = case shown="False" w571 {
                  tunnel: w588 -> [w625 _]
                  tunnel: w587 -> [w624 _]
                  tunnel: w586 -> [w623 _]
                  tunnel: w585 -> [w622 _]
                  tunnel: w584 -> [w621 _]
                  tunnel: w583 -> [w620 _]
                  tunnel: w582 -> [w619 _]
                  tunnel: w581 -> [w618 _]
                  tunnel: w573 -> [w617 _]
                  tunnel: w580 -> [w616 _]
                  tunnel: [w615 w626] -> w575
                  tunnel: w576 -> [w602 _]
                  tunnel: w574 -> [_ w626]
                  tunnel: w570 -> [_ _]
                  tunnel: w569 -> [w593 _]
                  tunnel: w568 -> [w591 _]
                  tunnel: w567 -> [w590 _]
                  tunnel: w566 -> [w589 _]
                  frame False {
                    # "dt = t2 -t1"
                    n207 = call "GetTimeInSeconds.vi"("Timestamp"=w602) -> ("Numeric"=w596:dbl)  [unwired: 10 in]
                    n208 = feedback-in #23(w596) -> ()
                    n209 = feedback #23(0.0 ("Numeric")) -> (w595:dbl)
                    n210 = Index Array(array=w617) -> (element #1=w604:dbl[], element #2=w607:dbl[])  [unwired: 4 in]
                    n211 = Subtract(x=w596, y=w595) -> (x-y=w598:dbl)
                    n212 = Empty Array?(array=w604) -> (empty?=w605:bool)
                    n213 = feedback #24(0.015 ("Numeric")) -> (w597:dbl)
                    n214 = Select(t=w616, s=w605, f=w604) -> (s? t:f=w603:dbl[])
                    n215 = Empty Array?(array=w607) -> (empty?=w608:bool)
                    n216 = Equal?(x=w598, y=0.0) -> (x = y?=w601:bool)
                    n217 = Select(t=w603, s=w608, f=w607) -> (s? t:f=w606:dbl[])
                    n218 = Select(t=w597, s=w601, f=w598) -> (s? t:f=w592:dbl)
                    n219 = call "PathVelocityProfile.vi"("Pose"=w616, "time"=w596, "intervalo"=w592, "estimatives"=w619, "Path  Smooth"=w617, "V_max"=w625, "Accel"=w624, "DesAccel"=w623) -> ("Time X"=w614:dbl[], "Velocities X"=w613:dbl[], "Time Y"=w612:dbl[], "Velocities Y"=w611:dbl[])  [unwired: 4 in]
                    n220 = call "VelocityCommand.vi"("intervalo"=w592, "MaxOutputXY"=w591, "estimatives"=w619, "Velocities Y"=w611, "Time Y"=w612, "Velocities X"=w613, "Time X"=w614) -> ("Vy"=w610:dbl, "Vx"=w609:dbl)  [unwired: 3 in]
                    n221 = feedback-in #24(w592) -> ()
                    n222 = call "VelocityControl.vi"("estimatives"=w619, "Vx"=w609, "PID Gains lateral"=w589, "Vy"=w610, "output xy"=w620, "Dest_orientation"=w618, "output inc"=w622, "PID Gains Angle"=w590, "Position"=w616, "output angle"=w621, "Waypoint 1"=w606, "PID gains Vel"=w593, "Waypoint 0"=w603) -> ("Output Velocity"=w615:dbl[])  [unwired: 6 in]
                  }
                  frame True {
                  }
                }
                n223 = feedback-in #22(w575) -> ()
                n224 = Index Array(array=w574) -> (element #1=w579:dbl, element #2=w578:dbl, element #3=w577:dbl)  [unwired: 3 in]
              }
              frame 8 {
                n225 = Not A Number/Path/Refnum?(number/path/refnum=w634) -> (NaN/Path/Refnum?=w633:bool[][])
                n226 = Or Array Elements(Boolean array=w633) -> (logical OR=w632:bool)
                n227 = feedback #25() -> (w635:dbl[])  [unwired: 1 in]
                n228 = case shown="False" w632 {
                  tunnel: w649 -> [w686 _]
                  tunnel: w648 -> [w685 _]
                  tunnel: w647 -> [w684 _]
                  tunnel: w646 -> [w683 _]
                  tunnel: w645 -> [w682 _]
                  tunnel: w644 -> [w681 _]
                  tunnel: w643 -> [w680 _]
                  tunnel: w642 -> [w679 _]
                  tunnel: w634 -> [w678 _]
                  tunnel: w641 -> [w677 _]
                  tunnel: [w676 w687] -> w636
                  tunnel: w637 -> [w663 _]
                  tunnel: w635 -> [_ w687]
                  tunnel: w631 -> [_ _]
                  tunnel: w630 -> [w654 _]
                  tunnel: w629 -> [w652 _]
                  tunnel: w628 -> [w651 _]
                  tunnel: w627 -> [w650 _]
                  frame False {
                    # "dt = t2 -t1"
                    n229 = call "GetTimeInSeconds.vi"("Timestamp"=w663) -> ("Numeric"=w657:dbl)  [unwired: 10 in]
                    n230 = feedback-in #26(w657) -> ()
                    n231 = feedback #26(0.0 ("Numeric")) -> (w656:dbl)
                    n232 = Index Array(array=w678) -> (element #1=w665:dbl[], element #2=w668:dbl[])  [unwired: 4 in]
                    n233 = Subtract(x=w657, y=w656) -> (x-y=w659:dbl)
                    n234 = Empty Array?(array=w665) -> (empty?=w666:bool)
                    n235 = feedback #27(0.015 ("Numeric")) -> (w658:dbl)
                    n236 = Select(t=w677, s=w666, f=w665) -> (s? t:f=w664:dbl[])
                    n237 = Empty Array?(array=w668) -> (empty?=w669:bool)
                    n238 = Equal?(x=w659, y=0.0) -> (x = y?=w662:bool)
                    n239 = Select(t=w664, s=w669, f=w668) -> (s? t:f=w667:dbl[])
                    n240 = Select(t=w658, s=w662, f=w659) -> (s? t:f=w653:dbl)
                    n241 = call "PathVelocityProfile.vi"("Pose"=w677, "time"=w657, "intervalo"=w653, "estimatives"=w680, "Path  Smooth"=w678, "V_max"=w686, "Accel"=w685, "DesAccel"=w684) -> ("Time X"=w675:dbl[], "Velocities X"=w674:dbl[], "Time Y"=w673:dbl[], "Velocities Y"=w672:dbl[])  [unwired: 4 in]
                    n242 = call "VelocityCommand.vi"("intervalo"=w653, "MaxOutputXY"=w652, "estimatives"=w680, "Velocities Y"=w672, "Time Y"=w673, "Velocities X"=w674, "Time X"=w675) -> ("Vy"=w671:dbl, "Vx"=w670:dbl)  [unwired: 3 in]
                    n243 = feedback-in #27(w653) -> ()
                    n244 = call "VelocityControl.vi"("estimatives"=w680, "Vx"=w670, "PID Gains lateral"=w650, "Vy"=w671, "output xy"=w681, "Dest_orientation"=w679, "output inc"=w683, "PID Gains Angle"=w651, "Position"=w677, "output angle"=w682, "Waypoint 1"=w667, "PID gains Vel"=w654, "Waypoint 0"=w664) -> ("Output Velocity"=w676:dbl[])  [unwired: 6 in]
                  }
                  frame True {
                  }
                }
                n245 = feedback-in #25(w636) -> ()
                n246 = Index Array(array=w635) -> (element #1=w640:dbl, element #2=w639:dbl, element #3=w638:dbl)  [unwired: 3 in]
              }
              frame 9 {
                n247 = Not A Number/Path/Refnum?(number/path/refnum=w695) -> (NaN/Path/Refnum?=w694:bool[][])
                n248 = Or Array Elements(Boolean array=w694) -> (logical OR=w693:bool)
                n249 = feedback #28() -> (w696:dbl[])  [unwired: 1 in]
                n250 = case shown="False" w693 {
                  tunnel: w710 -> [w747 _]
                  tunnel: w709 -> [w746 _]
                  tunnel: w708 -> [w745 _]
                  tunnel: w707 -> [w744 _]
                  tunnel: w706 -> [w743 _]
                  tunnel: w705 -> [w742 _]
                  tunnel: w704 -> [w741 _]
                  tunnel: w703 -> [w740 _]
                  tunnel: w695 -> [w739 _]
                  tunnel: w702 -> [w738 _]
                  tunnel: [w737 w748] -> w697
                  tunnel: w698 -> [w724 _]
                  tunnel: w696 -> [_ w748]
                  tunnel: w692 -> [_ _]
                  tunnel: w691 -> [w715 _]
                  tunnel: w690 -> [w713 _]
                  tunnel: w689 -> [w712 _]
                  tunnel: w688 -> [w711 _]
                  frame False {
                    # "dt = t2 -t1"
                    n251 = call "GetTimeInSeconds.vi"("Timestamp"=w724) -> ("Numeric"=w718:dbl)  [unwired: 10 in]
                    n252 = feedback-in #29(w718) -> ()
                    n253 = feedback #29(0.0 ("Numeric")) -> (w717:dbl)
                    n254 = Index Array(array=w739) -> (element #1=w726:dbl[], element #2=w729:dbl[])  [unwired: 4 in]
                    n255 = Subtract(x=w718, y=w717) -> (x-y=w720:dbl)
                    n256 = Empty Array?(array=w726) -> (empty?=w727:bool)
                    n257 = feedback #30(0.015 ("Numeric")) -> (w719:dbl)
                    n258 = Select(t=w738, s=w727, f=w726) -> (s? t:f=w725:dbl[])
                    n259 = Empty Array?(array=w729) -> (empty?=w730:bool)
                    n260 = Equal?(x=w720, y=0.0) -> (x = y?=w723:bool)
                    n261 = Select(t=w725, s=w730, f=w729) -> (s? t:f=w728:dbl[])
                    n262 = Select(t=w719, s=w723, f=w720) -> (s? t:f=w714:dbl)
                    n263 = call "PathVelocityProfile.vi"("Pose"=w738, "time"=w718, "intervalo"=w714, "estimatives"=w741, "Path  Smooth"=w739, "V_max"=w747, "Accel"=w746, "DesAccel"=w745) -> ("Time X"=w736:dbl[], "Velocities X"=w735:dbl[], "Time Y"=w734:dbl[], "Velocities Y"=w733:dbl[])  [unwired: 4 in]
                    n264 = call "VelocityCommand.vi"("intervalo"=w714, "MaxOutputXY"=w713, "estimatives"=w741, "Velocities Y"=w733, "Time Y"=w734, "Velocities X"=w735, "Time X"=w736) -> ("Vy"=w732:dbl, "Vx"=w731:dbl)  [unwired: 3 in]
                    n265 = feedback-in #30(w714) -> ()
                    n266 = call "VelocityControl.vi"("estimatives"=w741, "Vx"=w731, "PID Gains lateral"=w711, "Vy"=w732, "output xy"=w742, "Dest_orientation"=w740, "output inc"=w744, "PID Gains Angle"=w712, "Position"=w738, "output angle"=w743, "Waypoint 1"=w728, "PID gains Vel"=w715, "Waypoint 0"=w725) -> ("Output Velocity"=w737:dbl[])  [unwired: 6 in]
                  }
                  frame True {
                  }
                }
                n267 = feedback-in #28(w697) -> ()
                n268 = Index Array(array=w696) -> (element #1=w701:dbl, element #2=w700:dbl, element #3=w699:dbl)  [unwired: 3 in]
              }
              frame 10 {
                n269 = Not A Number/Path/Refnum?(number/path/refnum=w756) -> (NaN/Path/Refnum?=w755:bool[][])
                n270 = Or Array Elements(Boolean array=w755) -> (logical OR=w754:bool)
                n271 = feedback #31() -> (w757:dbl[])  [unwired: 1 in]
                n272 = case shown="False" w754 {
                  tunnel: w771 -> [w808 _]
                  tunnel: w770 -> [w807 _]
                  tunnel: w769 -> [w806 _]
                  tunnel: w768 -> [w805 _]
                  tunnel: w767 -> [w804 _]
                  tunnel: w766 -> [w803 _]
                  tunnel: w765 -> [w802 _]
                  tunnel: w764 -> [w801 _]
                  tunnel: w756 -> [w800 _]
                  tunnel: w763 -> [w799 _]
                  tunnel: [w798 w809] -> w758
                  tunnel: w759 -> [w785 _]
                  tunnel: w757 -> [_ w809]
                  tunnel: w753 -> [_ _]
                  tunnel: w752 -> [w776 _]
                  tunnel: w751 -> [w774 _]
                  tunnel: w750 -> [w773 _]
                  tunnel: w749 -> [w772 _]
                  frame False {
                    # "dt = t2 -t1"
                    n273 = call "GetTimeInSeconds.vi"("Timestamp"=w785) -> ("Numeric"=w779:dbl)  [unwired: 10 in]
                    n274 = feedback-in #32(w779) -> ()
                    n275 = feedback #32(0.0 ("Numeric")) -> (w778:dbl)
                    n276 = Index Array(array=w800) -> (element #1=w787:dbl[], element #2=w790:dbl[])  [unwired: 4 in]
                    n277 = Subtract(x=w779, y=w778) -> (x-y=w781:dbl)
                    n278 = Empty Array?(array=w787) -> (empty?=w788:bool)
                    n279 = feedback #33(0.015 ("Numeric")) -> (w780:dbl)
                    n280 = Select(t=w799, s=w788, f=w787) -> (s? t:f=w786:dbl[])
                    n281 = Empty Array?(array=w790) -> (empty?=w791:bool)
                    n282 = Equal?(x=w781, y=0.0) -> (x = y?=w784:bool)
                    n283 = Select(t=w786, s=w791, f=w790) -> (s? t:f=w789:dbl[])
                    n284 = Select(t=w780, s=w784, f=w781) -> (s? t:f=w775:dbl)
                    n285 = call "PathVelocityProfile.vi"("Pose"=w799, "time"=w779, "intervalo"=w775, "estimatives"=w802, "Path  Smooth"=w800, "V_max"=w808, "Accel"=w807, "DesAccel"=w806) -> ("Time X"=w797:dbl[], "Velocities X"=w796:dbl[], "Time Y"=w795:dbl[], "Velocities Y"=w794:dbl[])  [unwired: 4 in]
                    n286 = call "VelocityCommand.vi"("intervalo"=w775, "MaxOutputXY"=w774, "estimatives"=w802, "Velocities Y"=w794, "Time Y"=w795, "Velocities X"=w796, "Time X"=w797) -> ("Vy"=w793:dbl, "Vx"=w792:dbl)  [unwired: 3 in]
                    n287 = feedback-in #33(w775) -> ()
                    n288 = call "VelocityControl.vi"("estimatives"=w802, "Vx"=w792, "PID Gains lateral"=w772, "Vy"=w793, "output xy"=w803, "Dest_orientation"=w801, "output inc"=w805, "PID Gains Angle"=w773, "Position"=w799, "output angle"=w804, "Waypoint 1"=w789, "PID gains Vel"=w776, "Waypoint 0"=w786) -> ("Output Velocity"=w798:dbl[])  [unwired: 6 in]
                  }
                  frame True {
                  }
                }
                n289 = feedback-in #31(w758) -> ()
                n290 = Index Array(array=w757) -> (element #1=w762:dbl, element #2=w761:dbl, element #3=w760:dbl)  [unwired: 3 in]
              }
              frame 11 {
                n291 = Not A Number/Path/Refnum?(number/path/refnum=w817) -> (NaN/Path/Refnum?=w816:bool[][])
                n292 = Or Array Elements(Boolean array=w816) -> (logical OR=w815:bool)
                n293 = feedback #34() -> (w818:dbl[])  [unwired: 1 in]
                n294 = case shown="False" w815 {
                  tunnel: w832 -> [w869 _]
                  tunnel: w831 -> [w868 _]
                  tunnel: w830 -> [w867 _]
                  tunnel: w829 -> [w866 _]
                  tunnel: w828 -> [w865 _]
                  tunnel: w827 -> [w864 _]
                  tunnel: w826 -> [w863 _]
                  tunnel: w825 -> [w862 _]
                  tunnel: w817 -> [w861 _]
                  tunnel: w824 -> [w860 _]
                  tunnel: [w859 w870] -> w819
                  tunnel: w820 -> [w846 _]
                  tunnel: w818 -> [_ w870]
                  tunnel: w814 -> [_ _]
                  tunnel: w813 -> [w837 _]
                  tunnel: w812 -> [w835 _]
                  tunnel: w811 -> [w834 _]
                  tunnel: w810 -> [w833 _]
                  frame False {
                    # "dt = t2 -t1"
                    n295 = call "GetTimeInSeconds.vi"("Timestamp"=w846) -> ("Numeric"=w840:dbl)  [unwired: 10 in]
                    n296 = feedback-in #35(w840) -> ()
                    n297 = feedback #35(0.0 ("Numeric")) -> (w839:dbl)
                    n298 = Index Array(array=w861) -> (element #1=w848:dbl[], element #2=w851:dbl[])  [unwired: 4 in]
                    n299 = Subtract(x=w840, y=w839) -> (x-y=w842:dbl)
                    n300 = Empty Array?(array=w848) -> (empty?=w849:bool)
                    n301 = feedback #36(0.015 ("Numeric")) -> (w841:dbl)
                    n302 = Select(t=w860, s=w849, f=w848) -> (s? t:f=w847:dbl[])
                    n303 = Empty Array?(array=w851) -> (empty?=w852:bool)
                    n304 = Equal?(x=w842, y=0.0) -> (x = y?=w845:bool)
                    n305 = Select(t=w847, s=w852, f=w851) -> (s? t:f=w850:dbl[])
                    n306 = Select(t=w841, s=w845, f=w842) -> (s? t:f=w836:dbl)
                    n307 = call "PathVelocityProfile.vi"("Pose"=w860, "time"=w840, "intervalo"=w836, "estimatives"=w863, "Path  Smooth"=w861, "V_max"=w869, "Accel"=w868, "DesAccel"=w867) -> ("Time X"=w858:dbl[], "Velocities X"=w857:dbl[], "Time Y"=w856:dbl[], "Velocities Y"=w855:dbl[])  [unwired: 4 in]
                    n308 = call "VelocityCommand.vi"("intervalo"=w836, "MaxOutputXY"=w835, "estimatives"=w863, "Velocities Y"=w855, "Time Y"=w856, "Velocities X"=w857, "Time X"=w858) -> ("Vy"=w854:dbl, "Vx"=w853:dbl)  [unwired: 3 in]
                    n309 = feedback-in #36(w836) -> ()
                    n310 = call "VelocityControl.vi"("estimatives"=w863, "Vx"=w853, "PID Gains lateral"=w833, "Vy"=w854, "output xy"=w864, "Dest_orientation"=w862, "output inc"=w866, "PID Gains Angle"=w834, "Position"=w860, "output angle"=w865, "Waypoint 1"=w850, "PID gains Vel"=w837, "Waypoint 0"=w847) -> ("Output Velocity"=w859:dbl[])  [unwired: 6 in]
                  }
                  frame True {
                  }
                }
                n311 = feedback-in #34(w819) -> ()
                n312 = Index Array(array=w818) -> (element #1=w823:dbl, element #2=w822:dbl, element #3=w821:dbl)  [unwired: 3 in]
              }
              frame 12 {
                n313 = Not A Number/Path/Refnum?(number/path/refnum=w878) -> (NaN/Path/Refnum?=w877:bool[][])
                n314 = Or Array Elements(Boolean array=w877) -> (logical OR=w876:bool)
                n315 = feedback #37() -> (w879:dbl[])  [unwired: 1 in]
                n316 = case shown="False" w876 {
                  tunnel: w893 -> [w930 _]
                  tunnel: w892 -> [w929 _]
                  tunnel: w891 -> [w928 _]
                  tunnel: w890 -> [w927 _]
                  tunnel: w889 -> [w926 _]
                  tunnel: w888 -> [w925 _]
                  tunnel: w887 -> [w924 _]
                  tunnel: w886 -> [w923 _]
                  tunnel: w878 -> [w922 _]
                  tunnel: w885 -> [w921 _]
                  tunnel: [w920 w931] -> w880
                  tunnel: w881 -> [w907 _]
                  tunnel: w879 -> [_ w931]
                  tunnel: w875 -> [_ _]
                  tunnel: w874 -> [w898 _]
                  tunnel: w873 -> [w896 _]
                  tunnel: w872 -> [w895 _]
                  tunnel: w871 -> [w894 _]
                  frame False {
                    # "dt = t2 -t1"
                    n317 = call "GetTimeInSeconds.vi"("Timestamp"=w907) -> ("Numeric"=w901:dbl)  [unwired: 10 in]
                    n318 = feedback-in #38(w901) -> ()
                    n319 = feedback #38(0.0 ("Numeric")) -> (w900:dbl)
                    n320 = Index Array(array=w922) -> (element #1=w909:dbl[], element #2=w912:dbl[])  [unwired: 4 in]
                    n321 = Subtract(x=w901, y=w900) -> (x-y=w903:dbl)
                    n322 = Empty Array?(array=w909) -> (empty?=w910:bool)
                    n323 = feedback #39(0.015 ("Numeric")) -> (w902:dbl)
                    n324 = Select(t=w921, s=w910, f=w909) -> (s? t:f=w908:dbl[])
                    n325 = Empty Array?(array=w912) -> (empty?=w913:bool)
                    n326 = Equal?(x=w903, y=0.0) -> (x = y?=w906:bool)
                    n327 = Select(t=w908, s=w913, f=w912) -> (s? t:f=w911:dbl[])
                    n328 = Select(t=w902, s=w906, f=w903) -> (s? t:f=w897:dbl)
                    n329 = call "PathVelocityProfile.vi"("Pose"=w921, "time"=w901, "intervalo"=w897, "estimatives"=w924, "Path  Smooth"=w922, "V_max"=w930, "Accel"=w929, "DesAccel"=w928) -> ("Time X"=w919:dbl[], "Velocities X"=w918:dbl[], "Time Y"=w917:dbl[], "Velocities Y"=w916:dbl[])  [unwired: 4 in]
                    n330 = call "VelocityCommand.vi"("intervalo"=w897, "MaxOutputXY"=w896, "estimatives"=w924, "Velocities Y"=w916, "Time Y"=w917, "Velocities X"=w918, "Time X"=w919) -> ("Vy"=w915:dbl, "Vx"=w914:dbl)  [unwired: 3 in]
                    n331 = feedback-in #39(w897) -> ()
                    n332 = call "VelocityControl.vi"("estimatives"=w924, "Vx"=w914, "PID Gains lateral"=w894, "Vy"=w915, "output xy"=w925, "Dest_orientation"=w923, "output inc"=w927, "PID Gains Angle"=w895, "Position"=w921, "output angle"=w926, "Waypoint 1"=w911, "PID gains Vel"=w898, "Waypoint 0"=w908) -> ("Output Velocity"=w920:dbl[])  [unwired: 6 in]
                  }
                  frame True {
                  }
                }
                n333 = feedback-in #37(w880) -> ()
                n334 = Index Array(array=w879) -> (element #1=w884:dbl, element #2=w883:dbl, element #3=w882:dbl)  [unwired: 3 in]
              }
              frame 13 {
                n335 = Not A Number/Path/Refnum?(number/path/refnum=w939) -> (NaN/Path/Refnum?=w938:bool[][])
                n336 = Or Array Elements(Boolean array=w938) -> (logical OR=w937:bool)
                n337 = feedback #40() -> (w940:dbl[])  [unwired: 1 in]
                n338 = case shown="False" w937 {
                  tunnel: w954 -> [w991 _]
                  tunnel: w953 -> [w990 _]
                  tunnel: w952 -> [w989 _]
                  tunnel: w951 -> [w988 _]
                  tunnel: w950 -> [w987 _]
                  tunnel: w949 -> [w986 _]
                  tunnel: w948 -> [w985 _]
                  tunnel: w947 -> [w984 _]
                  tunnel: w939 -> [w983 _]
                  tunnel: w946 -> [w982 _]
                  tunnel: [w981 w992] -> w941
                  tunnel: w942 -> [w968 _]
                  tunnel: w940 -> [_ w992]
                  tunnel: w936 -> [_ _]
                  tunnel: w935 -> [w959 _]
                  tunnel: w934 -> [w957 _]
                  tunnel: w933 -> [w956 _]
                  tunnel: w932 -> [w955 _]
                  frame False {
                    # "dt = t2 -t1"
                    n339 = call "GetTimeInSeconds.vi"("Timestamp"=w968) -> ("Numeric"=w962:dbl)  [unwired: 10 in]
                    n340 = feedback-in #41(w962) -> ()
                    n341 = feedback #41(0.0 ("Numeric")) -> (w961:dbl)
                    n342 = Index Array(array=w983) -> (element #1=w970:dbl[], element #2=w973:dbl[])  [unwired: 4 in]
                    n343 = Subtract(x=w962, y=w961) -> (x-y=w964:dbl)
                    n344 = Empty Array?(array=w970) -> (empty?=w971:bool)
                    n345 = feedback #42(0.015 ("Numeric")) -> (w963:dbl)
                    n346 = Select(t=w982, s=w971, f=w970) -> (s? t:f=w969:dbl[])
                    n347 = Empty Array?(array=w973) -> (empty?=w974:bool)
                    n348 = Equal?(x=w964, y=0.0) -> (x = y?=w967:bool)
                    n349 = Select(t=w969, s=w974, f=w973) -> (s? t:f=w972:dbl[])
                    n350 = Select(t=w963, s=w967, f=w964) -> (s? t:f=w958:dbl)
                    n351 = call "PathVelocityProfile.vi"("Pose"=w982, "time"=w962, "intervalo"=w958, "estimatives"=w985, "Path  Smooth"=w983, "V_max"=w991, "Accel"=w990, "DesAccel"=w989) -> ("Time X"=w980:dbl[], "Velocities X"=w979:dbl[], "Time Y"=w978:dbl[], "Velocities Y"=w977:dbl[])  [unwired: 4 in]
                    n352 = call "VelocityCommand.vi"("intervalo"=w958, "MaxOutputXY"=w957, "estimatives"=w985, "Velocities Y"=w977, "Time Y"=w978, "Velocities X"=w979, "Time X"=w980) -> ("Vy"=w976:dbl, "Vx"=w975:dbl)  [unwired: 3 in]
                    n353 = feedback-in #42(w958) -> ()
                    n354 = call "VelocityControl.vi"("estimatives"=w985, "Vx"=w975, "PID Gains lateral"=w955, "Vy"=w976, "output xy"=w986, "Dest_orientation"=w984, "output inc"=w988, "PID Gains Angle"=w956, "Position"=w982, "output angle"=w987, "Waypoint 1"=w972, "PID gains Vel"=w959, "Waypoint 0"=w969) -> ("Output Velocity"=w981:dbl[])  [unwired: 6 in]
                  }
                  frame True {
                  }
                }
                n355 = feedback-in #40(w941) -> ()
                n356 = Index Array(array=w940) -> (element #1=w945:dbl, element #2=w944:dbl, element #3=w943:dbl)  [unwired: 3 in]
              }
              frame 14 {
                n357 = Not A Number/Path/Refnum?(number/path/refnum=w1000) -> (NaN/Path/Refnum?=w999:bool[][])
                n358 = Or Array Elements(Boolean array=w999) -> (logical OR=w998:bool)
                n359 = feedback #43() -> (w1001:dbl[])  [unwired: 1 in]
                n360 = case shown="False" w998 {
                  tunnel: w1015 -> [w1052 _]
                  tunnel: w1014 -> [w1051 _]
                  tunnel: w1013 -> [w1050 _]
                  tunnel: w1012 -> [w1049 _]
                  tunnel: w1011 -> [w1048 _]
                  tunnel: w1010 -> [w1047 _]
                  tunnel: w1009 -> [w1046 _]
                  tunnel: w1008 -> [w1045 _]
                  tunnel: w1000 -> [w1044 _]
                  tunnel: w1007 -> [w1043 _]
                  tunnel: [w1042 w1053] -> w1002
                  tunnel: w1003 -> [w1029 _]
                  tunnel: w1001 -> [_ w1053]
                  tunnel: w997 -> [_ _]
                  tunnel: w996 -> [w1020 _]
                  tunnel: w995 -> [w1018 _]
                  tunnel: w994 -> [w1017 _]
                  tunnel: w993 -> [w1016 _]
                  frame False {
                    # "dt = t2 -t1"
                    n361 = call "GetTimeInSeconds.vi"("Timestamp"=w1029) -> ("Numeric"=w1023:dbl)  [unwired: 10 in]
                    n362 = feedback-in #44(w1023) -> ()
                    n363 = feedback #44(0.0 ("Numeric")) -> (w1022:dbl)
                    n364 = Index Array(array=w1044) -> (element #1=w1031:dbl[], element #2=w1034:dbl[])  [unwired: 4 in]
                    n365 = Subtract(x=w1023, y=w1022) -> (x-y=w1025:dbl)
                    n366 = Empty Array?(array=w1031) -> (empty?=w1032:bool)
                    n367 = feedback #45(0.015 ("Numeric")) -> (w1024:dbl)
                    n368 = Select(t=w1043, s=w1032, f=w1031) -> (s? t:f=w1030:dbl[])
                    n369 = Empty Array?(array=w1034) -> (empty?=w1035:bool)
                    n370 = Equal?(x=w1025, y=0.0) -> (x = y?=w1028:bool)
                    n371 = Select(t=w1030, s=w1035, f=w1034) -> (s? t:f=w1033:dbl[])
                    n372 = Select(t=w1024, s=w1028, f=w1025) -> (s? t:f=w1019:dbl)
                    n373 = call "PathVelocityProfile.vi"("Pose"=w1043, "time"=w1023, "intervalo"=w1019, "estimatives"=w1046, "Path  Smooth"=w1044, "V_max"=w1052, "Accel"=w1051, "DesAccel"=w1050) -> ("Time X"=w1041:dbl[], "Velocities X"=w1040:dbl[], "Time Y"=w1039:dbl[], "Velocities Y"=w1038:dbl[])  [unwired: 4 in]
                    n374 = call "VelocityCommand.vi"("intervalo"=w1019, "MaxOutputXY"=w1018, "estimatives"=w1046, "Velocities Y"=w1038, "Time Y"=w1039, "Velocities X"=w1040, "Time X"=w1041) -> ("Vy"=w1037:dbl, "Vx"=w1036:dbl)  [unwired: 3 in]
                    n375 = feedback-in #45(w1019) -> ()
                    n376 = call "VelocityControl.vi"("estimatives"=w1046, "Vx"=w1036, "PID Gains lateral"=w1016, "Vy"=w1037, "output xy"=w1047, "Dest_orientation"=w1045, "output inc"=w1049, "PID Gains Angle"=w1017, "Position"=w1043, "output angle"=w1048, "Waypoint 1"=w1033, "PID gains Vel"=w1020, "Waypoint 0"=w1030) -> ("Output Velocity"=w1042:dbl[])  [unwired: 6 in]
                  }
                  frame True {
                  }
                }
                n377 = feedback-in #43(w1002) -> ()
                n378 = Index Array(array=w1001) -> (element #1=w1006:dbl, element #2=w1005:dbl, element #3=w1004:dbl)  [unwired: 3 in]
              }
              frame 15 {
                n379 = Not A Number/Path/Refnum?(number/path/refnum=w1061) -> (NaN/Path/Refnum?=w1060:bool[][])
                n380 = Or Array Elements(Boolean array=w1060) -> (logical OR=w1059:bool)
                n381 = feedback #46() -> (w1062:dbl[])  [unwired: 1 in]
                n382 = case shown="False" w1059 {
                  tunnel: w1076 -> [w1113 _]
                  tunnel: w1075 -> [w1112 _]
                  tunnel: w1074 -> [w1111 _]
                  tunnel: w1073 -> [w1110 _]
                  tunnel: w1072 -> [w1109 _]
                  tunnel: w1071 -> [w1108 _]
                  tunnel: w1070 -> [w1107 _]
                  tunnel: w1069 -> [w1106 _]
                  tunnel: w1061 -> [w1105 _]
                  tunnel: w1068 -> [w1104 _]
                  tunnel: [w1103 w1114] -> w1063
                  tunnel: w1064 -> [w1090 _]
                  tunnel: w1062 -> [_ w1114]
                  tunnel: w1058 -> [_ _]
                  tunnel: w1057 -> [w1081 _]
                  tunnel: w1056 -> [w1079 _]
                  tunnel: w1055 -> [w1078 _]
                  tunnel: w1054 -> [w1077 _]
                  frame False {
                    # "dt = t2 -t1"
                    n383 = call "GetTimeInSeconds.vi"("Timestamp"=w1090) -> ("Numeric"=w1084:dbl)  [unwired: 10 in]
                    n384 = feedback-in #47(w1084) -> ()
                    n385 = feedback #47(0.0 ("Numeric")) -> (w1083:dbl)
                    n386 = Index Array(array=w1105) -> (element #1=w1092:dbl[], element #2=w1095:dbl[])  [unwired: 4 in]
                    n387 = Subtract(x=w1084, y=w1083) -> (x-y=w1086:dbl)
                    n388 = Empty Array?(array=w1092) -> (empty?=w1093:bool)
                    n389 = feedback #48(0.015 ("Numeric")) -> (w1085:dbl)
                    n390 = Select(t=w1104, s=w1093, f=w1092) -> (s? t:f=w1091:dbl[])
                    n391 = Empty Array?(array=w1095) -> (empty?=w1096:bool)
                    n392 = Equal?(x=w1086, y=0.0) -> (x = y?=w1089:bool)
                    n393 = Select(t=w1091, s=w1096, f=w1095) -> (s? t:f=w1094:dbl[])
                    n394 = Select(t=w1085, s=w1089, f=w1086) -> (s? t:f=w1080:dbl)
                    n395 = call "PathVelocityProfile.vi"("Pose"=w1104, "time"=w1084, "intervalo"=w1080, "estimatives"=w1107, "Path  Smooth"=w1105, "V_max"=w1113, "Accel"=w1112, "DesAccel"=w1111) -> ("Time X"=w1102:dbl[], "Velocities X"=w1101:dbl[], "Time Y"=w1100:dbl[], "Velocities Y"=w1099:dbl[])  [unwired: 4 in]
                    n396 = call "VelocityCommand.vi"("intervalo"=w1080, "MaxOutputXY"=w1079, "estimatives"=w1107, "Velocities Y"=w1099, "Time Y"=w1100, "Velocities X"=w1101, "Time X"=w1102) -> ("Vy"=w1098:dbl, "Vx"=w1097:dbl)  [unwired: 3 in]
                    n397 = feedback-in #48(w1080) -> ()
                    n398 = call "VelocityControl.vi"("estimatives"=w1107, "Vx"=w1097, "PID Gains lateral"=w1077, "Vy"=w1098, "output xy"=w1108, "Dest_orientation"=w1106, "output inc"=w1110, "PID Gains Angle"=w1078, "Position"=w1104, "output angle"=w1109, "Waypoint 1"=w1094, "PID gains Vel"=w1081, "Waypoint 0"=w1091) -> ("Output Velocity"=w1103:dbl[])  [unwired: 6 in]
                  }
                  frame True {
                  }
                }
                n399 = feedback-in #46(w1063) -> ()
                n400 = Index Array(array=w1062) -> (element #1=w1067:dbl, element #2=w1066:dbl, element #3=w1065:dbl)  [unwired: 3 in]
              }
            }
          }
          frame True {
            w1115 = 0.0 ("output")
          }
        }
        n401 = Bundle By Name(cluster=w118, "v_tangent"=w104, "v_normal"=w103, "v_ang"=w99) -> (w117:T1)
      }
      n402 = Bundle By Name(cluster=w38, "our_robots"=w39) -> (w37:T14)
    }
    frame True {
      n403 = Unbundle By Name(w1119) -> ("our_robots"=w1120:T1[])
      n404 = for {
        tunnel: w1120 -> [w1138] mode=indexing
        tunnel: [w1133] -> w1118 mode=indexing
        tunnel: w1116 -> [w1132]
        w1123 = 1000.0 ("y")
        n405 = Unbundle By Name(w1138) -> ("x"=w1124:dbl, "y"=w1126:dbl, "orientation"=w1146:dbl, "Dest"=w1144:T5)
        n406 = Unbundle By Name(w1132) -> ("PID gains Angle GoTo"=w1127:cluster{"(Kc)":dbl, "(Ki)":dbl, "(Kd)":dbl}, "PID gains XY GoTo"=w1128:cluster{"(Kc)":dbl, "(Ki)":dbl, "(Kd)":dbl}, "Max Params GoTo"=w1131:T20)
        n407 = Index Array(array=w1144) -> (element=w1143:T6)  [unwired: 1 in]
        n408 = Divide(x=w1126, y=w1123) -> (x/y=w1125:dbl)
        n409 = Divide(x=w1124, y=w1123) -> (x/y=w1122:dbl)
        n410 = Unbundle By Name(w1131) -> ("Max output XY"=w1130:dbl, "MaxOutput Angle"=w1129:dbl)
        n411 = Build Array(w1122, w1125, w1146) -> (w1145:dbl[])
        n412 = Unbundle By Name(w1143) -> ("dest_x"=w1142:dbl, "dest_y"=w1141:dbl, "dest_orientation"=w1140:dbl)
        n413 = Build Array(w1142, w1141, w1140) -> (w1139:dbl[])
        n414 = call "GoTo.vi"("PID Gains Angle"=w1127, "PID Gains XY"=w1128, "output angle"=w1129, "output xy"=w1130, "Target"=w1139, "Position"=w1145) -> ("Output\nVelocity"=w1137:dbl[])  [unwired: 4 in, 1 out]
        n415 = Index Array(array=w1137) -> (element #1=w1136:dbl, element #2=w1135:dbl, element #3=w1134:dbl)  [unwired: 3 in]
        n416 = Bundle By Name(cluster=w1138, "v_tangent"=w1136, "v_normal"=w1135, "v_ang"=w1134) -> (w1133:T1)
      }
      n417 = Bundle By Name(cluster=w1119, "our_robots"=w1118) -> (w1117:T14)
      n418 = call "potential-field.vi"("IA State Output in"=w1117) -> ("IA State Output out"=w1121:T14)  [unwired: 10 in]
    }
  }
  n419 = Unbundle By Name(w9) -> ("IA Judge.command enum"=w8:T18)
  n420 = Equal?(x=w8, y=Command_Enum."Halt") -> (x = y?=w5:bool)
  n421 = Or(x="Debug", y=w5) -> (x .or. y?=w6:bool)
  n422 = case shown="True" w6 {
    tunnel: [w1147 w1152] -> w10
    tunnel: w9 -> [w1147 w1149]
    tunnel: "IA State Output in" -> [_ w1150]
    frame False {
    }
    frame True {
      n423 = Unbundle By Name(w1149) -> ("our_robots"=w1148:T1[])
      n424 = for {
        tunnel: [w1155] -> w1151 mode=indexing
        tunnel: w1148 -> [w1153] mode=indexing
        workers-P: _ -> [_]
        w1154 = 0.0 ("v_normal")
        n425 = Bundle By Name(cluster=w1153, "v_tangent"=w1154, "v_normal"=w1154, "v_ang"=w1154) -> (w1155:T1)
      }
      n426 = Bundle By Name(cluster=w1150, "our_robots"=w1151) -> (w1152:T14)
    }
  }
  "IA State Output out" <- w10
